vi "Vision_Left_MANUAL_RUN_R0.vi"() -> ()   [LabVIEW 2015]
uses:
  <vilib>/vision/Pattern Matching.llb/IMAQ Curve Parameters.ctl
  <vilib>/vision/Pattern Matching.llb/IMAQ Match Range Setting.ctl
  <vilib>/userdefined/High Color/IMAQdx.ctl
  <vilib>/vision/driver/NI_Vision_Acquisition_Software.lvlib
  <vilib>/vision/NI_Vision_Development_Module.lvlib
panel:
  in  "Range 0 Default\nSetting Values":T1={"Min Scale"=25.0, "Max Scale"=250.0, "Min Score"=850.0, "Lower Transition Scale"=1.0, "Upper Transition Scale"=200.0, "ROI Vertical"=2.0, "ROI Horizontal"=1.0, "Scale Cushion"=15.0, "Curve Parameters"={"Min Length"=15, "Row Search Step"=10, "Col Search Step"=10}, "Beacon Cushion (px)"=3.0, "Max Scale Diff\nfrom Main"=50.0}
  in  "Range 0 Templates":T2={"Sub - 2 File Path"=path "/home/lvuser/Beacon_Templates/Range_0/Range 0.png", "Sub Beacon Template File Path - ARRAY"=[path "/home/lvuser/Beacon_Templates/Range_1/Sub 0 - Range 1.png", path "/home/lvuser/Beacon_Templates/Range_1/Sub 1 - Range 1.png", path "/home/lvuser/Beacon_Templates/Range_1/Sub 2 - Range 1.png", path "/home/lvuser/Beacon_Templates/Range_1/Sub 3 - Range 1.png", path "/home/lvuser/Beacon_Templates/Range_1/Sub 4 - Range 1.png"]}
  in  "Correlation Score Threhsold (Range 0)":sgl=800.0
  in  "stop":bool
  in  "select (true= use advanced features\nfase= dont use)":bool
  in  "Range 3 Default\nSetting Values":T1={"Min Scale"=50.0, "Max Scale"=150.0, "Min Score"=800.0, "Lower Transition Scale"=1.0, "Upper Transition Scale"=120.0, "ROI Vertical"=3.5, "ROI Horizontal"=4.0, "Scale Cushion"=15.0, "Curve Parameters"={"Min Length"=3, "Row Search Step"=5, "Col Search Step"=5}, "Beacon Cushion (px)"=5.0, "Max Scale Diff\nfrom Main"=10.0}
  in  "Range 2 Default\nSetting Values":T1={"Min Scale"=65.0, "Max Scale"=130.0, "Min Score"=800.0, "Lower Transition Scale"=70.0, "Upper Transition Scale"=115.0, "ROI Vertical"=2.8, "ROI Horizontal"=4.0, "Scale Cushion"=2.0, "Curve Parameters"={"Min Length"=10, "Row Search Step"=10, "Col Search Step"=10}, "Beacon Cushion (px)"=15.0, "Max Scale Diff\nfrom Main"=20.0}
  in  "ROI Decay Factor (px)":dbl=50.0
  in  "ROBOT STATE\n(fwd, bwd, neither) 2":i32
  in  "Score Decay \nFactor 2":dbl=50.0
  in  "Range 1 Default\nSetting Values":T1={"Min Scale"=25.0, "Max Scale"=100.0, "Min Score"=800.0, "Lower Transition Scale"=35.0, "Upper Transition Scale"=67.0, "ROI Vertical"=0.75, "ROI Horizontal"=5.0, "Scale Cushion"=23.0, "Curve Parameters"={"Min Length"=15, "Row Search Step"=15, "Col Search Step"=15}, "Beacon Cushion (px)"=25.0, "Max Scale Diff\nfrom Main"=25.0}
  out "Next Template":T3(ring)=enum."Range 0"
  out "Current Template":T3(ring)=enum."Range 0"
  in  "Initial Template":T3(ring)=enum."Range 0"
  in  "Range 3 Templates":T2={"Sub - 2 File Path"=path "/home/lvuser/Beacon_Templates/Range_3/5 Beacons - Range 3.png", "Sub Beacon Template File Path - ARRAY"=[path "/home/lvuser/Beacon_Templates/Range_3/Sub 0 - Range 3.png", path "/home/lvuser/Beacon_Templates/Range_3/Sub 1 - Range 3.png", path "/home/lvuser/Beacon_Templates/Range_3/Sub 2 - Range 3.png", path "/home/lvuser/Beacon_Templates/Range_3/Sub 3 - Range 3.png", path "/home/lvuser/Beacon_Templates/Range_3/Sub 4 - Range 3.png"]}
  in  "Range 2 Templates":T2={"Sub - 2 File Path"=path "/home/lvuser/Beacon_Templates/Range_2/5 Beacons - Range 2.png", "Sub Beacon Template File Path - ARRAY"=[path "/home/lvuser/Beacon_Templates/Range_2/Sub 0 - Range 2.png", path "/home/lvuser/Beacon_Templates/Range_2/Sub 1 - Range 2.png", path "/home/lvuser/Beacon_Templates/Range_2/Sub 2 - Range 2.png", path "/home/lvuser/Beacon_Templates/Range_2/Sub 3 - Range 2.png", path "/home/lvuser/Beacon_Templates/Range_2/Sub 4 - Range 2.png"]}
  in  "Range 1 Templates - LEFT":T2={"Sub - 2 File Path"=path "/home/lvuser/Beacon_Templates/Range_1/2_Beacons_Left - Range 1.png", "Sub Beacon Template File Path - ARRAY"=[path "/home/lvuser/Beacon_Templates/Range_1/Sub 0 - Range 1.png", path "/home/lvuser/Beacon_Templates/Range_1/Sub 1 - Range 1.png", path "/home/lvuser/Beacon_Templates/Range_1/Sub 2 - Range 1.png", path "/home/lvuser/Beacon_Templates/Range_1/Sub 3 - Range 1.png", path "/home/lvuser/Beacon_Templates/Range_1/Sub 4 - Range 1.png"]}
  out "Current Correlation Score":sgl
  in  "Correlation Score Threhsold":sgl=300.0
  out "New Min Score":dbl=850.0
  out "New Low Scale":dbl=50.0
  out "New high Scale":dbl=250.0
  in  "Absolute\nMinimum Score":dbl=750.0
  in  "Absolute\nMaximum Scale":dbl=250.0
  in  "Absolute\nMinimum Scale":dbl=25.0
  in  "Score\nCushion":dbl=192.0
  in  "Avg Scale - Last":dbl=25.73214817047119
  in  "Avg Score - Last":dbl=994.8521728515625
  in  "Max Window\n for Avg":u8=3
  in  "Valid Treshold\nfor Lock":i16=3
  out "Current  Score":sgl
  out "Current  Scale":sgl
  out "Current Valid?":bool
  out "Beacon - Scales":sgl[](array[numeric])
  out "beacon - Scores":sgl[](array[numeric])
  out "Beacons Found":bool[](array[boolean])
  out "Horiztonall Beacon \nCushion (pixels)":sgl=15.0
  out "Tracking Info":T4={"Lock"=FALSE, "Current Valid"=FALSE, "Current Template"=enum."Range 0", "Tracking Coordinates"={"X"=159.0, "Y"=119.0}, "Setting Values"={"Min Score"=850.0, "Min Scale"=50.0, "Max Scale"=250.0, "Curve Parameters"={"Min Length"=15, "Row Search Step"=10, "Col Search Step"=10}}}
  out "dT":u32=467
  out "Avg Scale":dbl=25.73214817047119
  out "Avg Score":dbl=994.8521728515625
  out "Current Search Settings":T7={"Curve Parameters"={"Extraction Mode"=1, "Edge Threshold"=200, "Edge Filter Size"=0, "Min Length"=15, "Row Search Step Size"=10, "Col Search Step Size"=10, "Max Endpoint Gap"=4, "Closed"=TRUE, "Subpixel"=TRUE}, "Match Mode"={"Rotation"=FALSE, "Scale"=TRUE, "Occlusion"=TRUE, "Reserved"=FALSE, "Reserved"=FALSE, "Reserved"=FALSE}, "Range Settings"=[{"Match Constraints"=0, "Min"=-2.0, "Max"=2.0}, {"Match Constraints"=1, "Min"=50.0, "Max"=250.0}, {"Match Constraints"=2, "Min"=0.0, "Max"=20.0}], "Number of Matches"=1, "Minimum Match Score"=850.0, "SubPixel Accuracy"=TRUE, "Adv. Geometric Match Options 2"=[{"Setup Data Item"=20, "Item Value"=0.0}, {"Setup Data Item"=22, "Item Value"=1.0}]} {"Curve Parameters"."Extraction Mode" items=["Normal", "Uniform Regions"]; "Curve Parameters"."Edge Filter Size" items=["Fine", "Normal", "Contour Tracing"]; "Curve Parameters"."Max Endpoint Gap" min=0; "Curve Parameters"."Col Search Step Size" min=1 max=255 step=1; "Curve Parameters"."Row Search Step Size" min=1 max=255 step=1; "Curve Parameters"."Min Length" min=0; "Curve Parameters"."Edge Threshold" min=1 max=350 step=1; "Range Settings"."Max" format="%.2f"; "Range Settings"."Min" format="%.2f"; "Range Settings"."Match Constraints" items=["Rotation Angle (degrees)", "Scale Factor (%)", "Occlusion (%)"]}
  out "Valid Scale History":dbl[](array[numeric]) format="%#_13g"
  out "Valid Score History":dbl[](array[numeric]) format="%#_13g"
  out "Valid Beacon History - in":bool[](array[boolean])
  out "Startup Flag":bool
  out "Lock Status":bool
  out "Y Coordinates":sgl[](array[numeric])
  out "X Coordinates":sgl[](array[numeric])
  out "Right Image out":T8(plugin-control)
  in  "History Size":i32=20
  in  "INITIAL Search Settings":T7={"Curve Parameters"={"Extraction Mode"=1, "Edge Threshold"=200, "Edge Filter Size"=0, "Min Length"=15, "Row Search Step Size"=10, "Col Search Step Size"=10, "Max Endpoint Gap"=4, "Closed"=TRUE, "Subpixel"=TRUE}, "Match Mode"={"Rotation"=FALSE, "Scale"=TRUE, "Occlusion"=TRUE, "Reserved"=FALSE, "Reserved"=FALSE, "Reserved"=FALSE}, "Range Settings"=[{"Match Constraints"=0, "Min"=-2.0, "Max"=2.0}, {"Match Constraints"=1, "Min"=25.0, "Max"=250.0}, {"Match Constraints"=2, "Min"=0.0, "Max"=20.0}], "Number of Matches"=1, "Minimum Match Score"=800.0, "SubPixel Accuracy"=TRUE, "Adv. Geometric Match Options 2"=[{"Setup Data Item"=20, "Item Value"=0.0}, {"Setup Data Item"=22, "Item Value"=1.0}]} {"Curve Parameters"."Extraction Mode" items=["Normal", "Uniform Regions"]; "Curve Parameters"."Edge Filter Size" items=["Fine", "Normal", "Contour Tracing"]; "Curve Parameters"."Max Endpoint Gap" min=0; "Curve Parameters"."Col Search Step Size" min=1 max=255 step=1; "Curve Parameters"."Row Search Step Size" min=1 max=255 step=1; "Curve Parameters"."Min Length" min=0; "Curve Parameters"."Edge Threshold" min=1 max=350 step=1; "Range Settings"."Max" format="%.2f"; "Range Settings"."Min" format="%.2f"; "Range Settings"."Match Constraints" items=["Rotation Angle (degrees)", "Scale Factor (%)", "Occlusion (%)"]; "Adv. Geometric Match Options 2"."Setup Data Item" items=["Curve Extraction Mode", "Curve Edge Threshold", "Curve Edge Filter Size", "Min Curve Length", "Curve Row Search Step Size", "Curve Col Search Step Size", "Curve Max Endpoint Gap", "Extract Closed Curves", "Enable Subpixel Curve Extraction", "Enable Correlation Score", "Enable Subpixel Accuracy", "Subpixel Iterations", "Subpixel Tolerance", "Initial Match List Length", "Enable Target Template Curve Score", "Min Match Separation Distance", "Min Match Separation Angle", "Min Match Separation Scale", "Max Match Overlap", "Enable Coarse Result", "Enable Calibration Support", "Enable Contrast Reversal", "Search Strategy", "Refinement Match Factor", "Subpixel Match Factor"]}
  # "ROI Factore (per Template)"
  # "Template Transition Scales"
  # "Search Parameter Limits"
  # "TEMPLATE FILE PATHS"
  # "Config"
  # "Initial Settings"
  # "test"
  # "Range"
  # "Range"
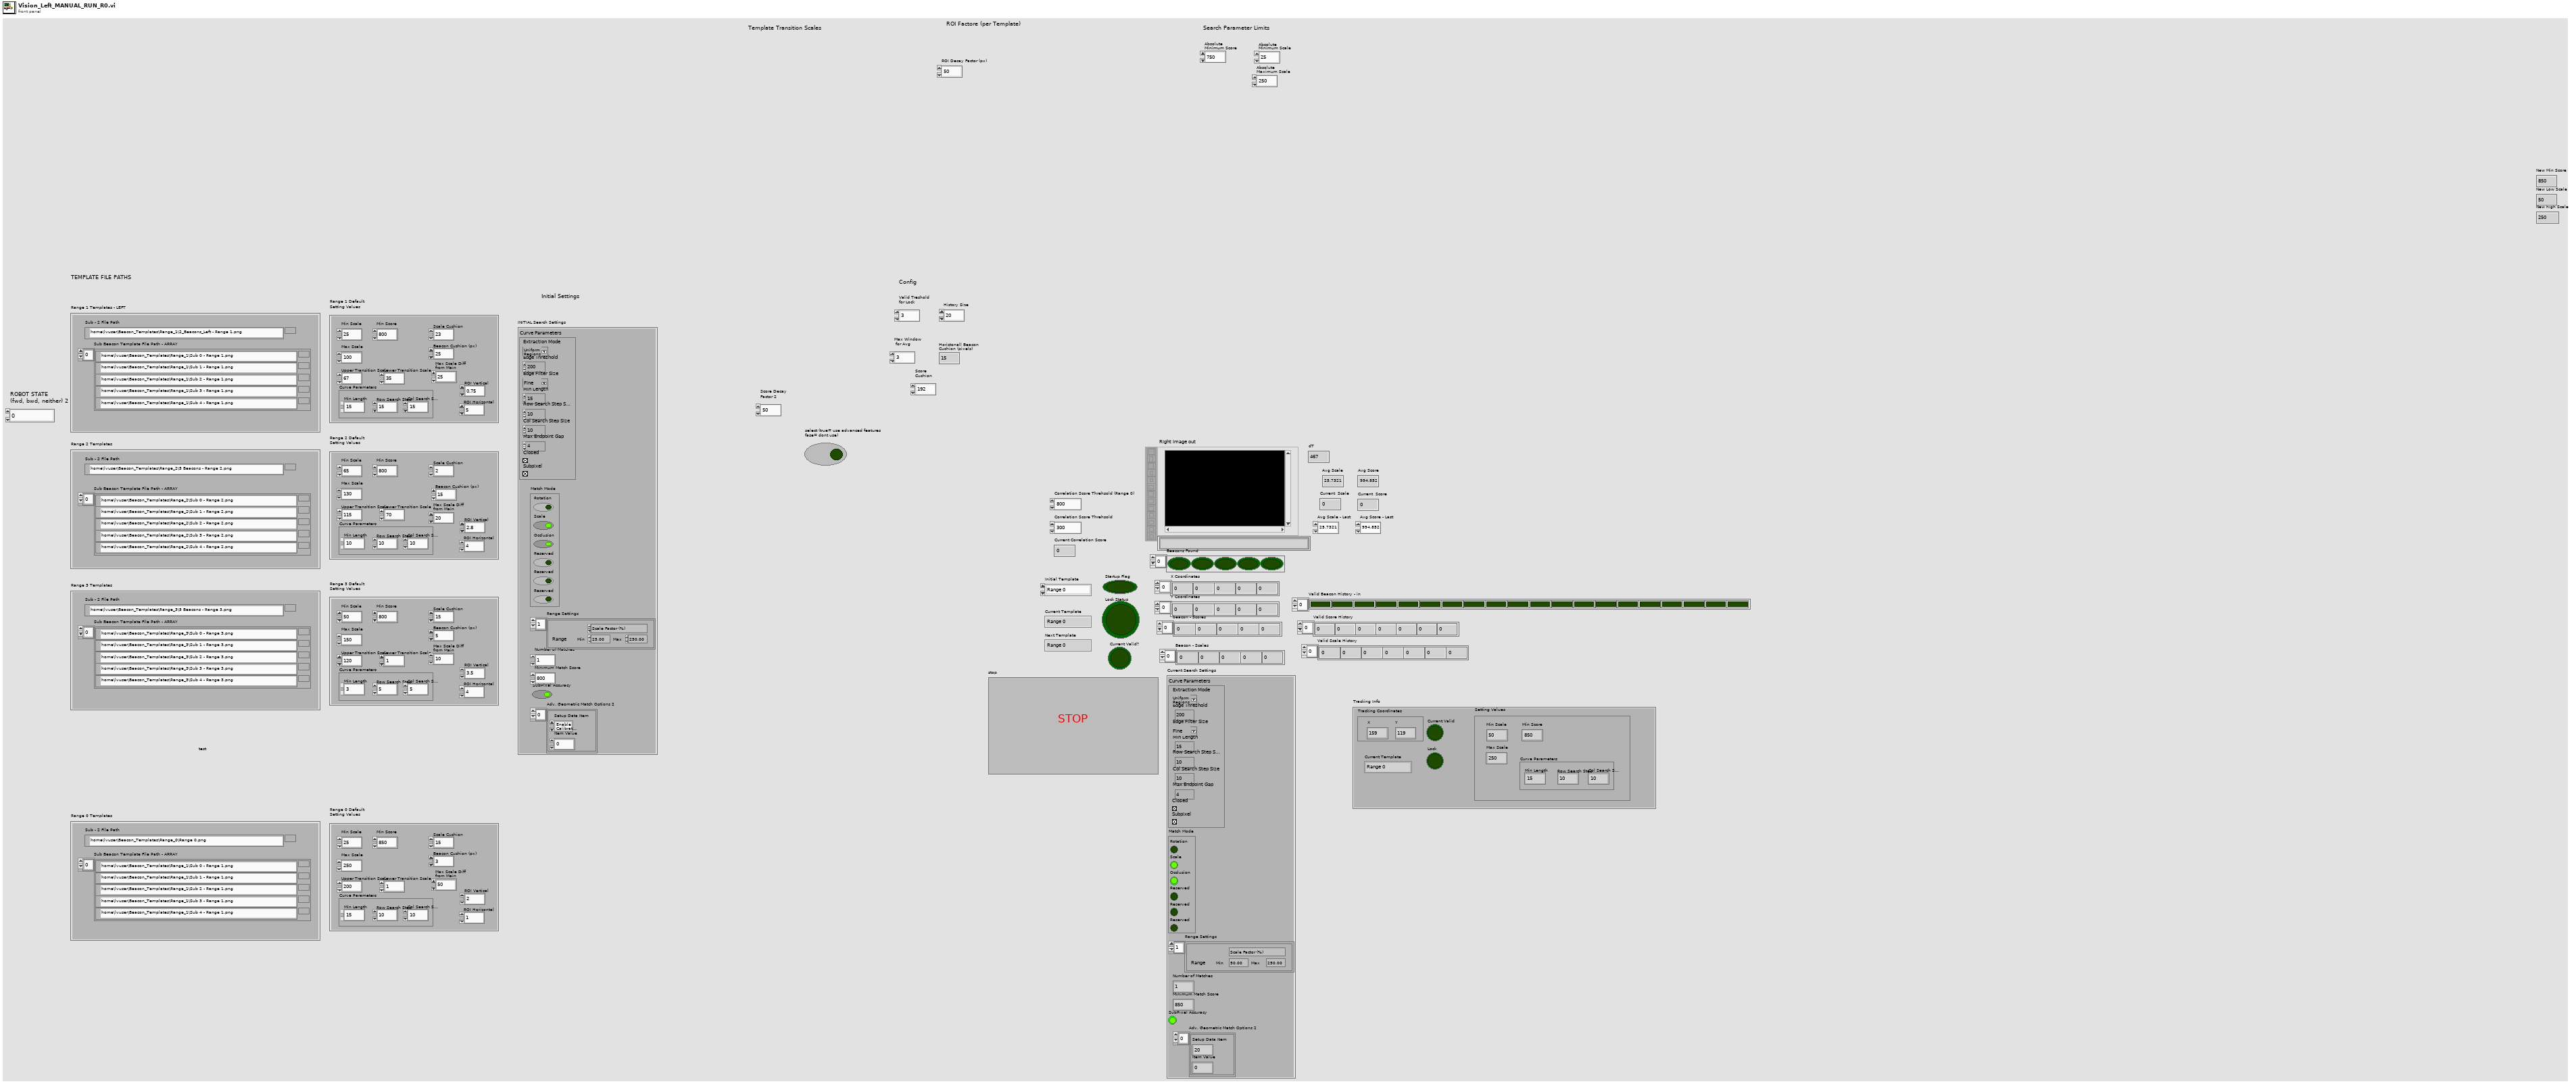
[diagram p1: front panel]
types:
  T1 = cluster{"Min Scale":dbl, "Max Scale":dbl, "Min Score":dbl, "Lower Transition Scale":sgl, "Upper Transition Scale":sgl, "ROI Vertical":dbl, "ROI Horizontal":dbl, "Scale Cushion":dbl, "Curve Parameters":cluster{"Min Length":i32, "Row Search Step":i32, "Col Search Step":i32}, "Beacon Cushion (px)":dbl, "Max Scale Diff\nfrom Main":dbl}
  T2 = cluster{"Sub - 2 File Path":path, "Sub Beacon Template File Path - ARRAY":path[]}
  T3 = enum16{"Range 1", "Range 2", "Range 3", "Range 0"}
  T4 = cluster{"Lock":bool, "Current Valid":bool, "Current Template":enum16{"Range 1", "Range 2", "Range 3", "Range 0"}, "Tracking Coordinates":cluster{"X":dbl, "Y":dbl}, "Setting Values":cluster{"Min Score":dbl, "Min Scale":dbl, "Max Scale":dbl, "Curve Parameters":cluster{"Min Length":i32, "Row Search Step":i32, "Col Search Step":i32}}}
  T5 = typedef "IMAQ Curve Parameters.ctl" = cluster{"Extraction Mode":u32, "Edge Threshold":i32, "Edge Filter Size":u32, "Min Length":i32, "Row Search Step Size":i32, "Col Search Step Size":i32, "Max Endpoint Gap":i32, "Closed":bool, "Subpixel":bool}
  T6 = typedef "IMAQ Match Range Setting.ctl" = cluster{"Match Constraints":u32, "Min":dbl, "Max":dbl}
  T7 = cluster{"Curve Parameters":T5, "Match Mode":cluster{"Rotation":bool, "Scale":bool, "Occlusion":bool, "Reserved":bool, "Reserved":bool, "Reserved":bool}, "Range Settings":T6[], "Number of Matches":i32, "Minimum Match Score":sgl, "SubPixel Accuracy":bool, "Adv. Geometric Match Options 2":cluster{"Setup Data Item":u16, "Item Value":dbl}[]}
  T8 = typedef "IMAQ Image.ctl" = refnum<image>
  T9 = typedef "IMAQdx.ctl" = refnum<k21>
  T10 = typedef "Image Type" = u32
  T11 = typedef "ROI Descriptor" = cluster{"Global Rectangle":i32[], "Contours":cluster{"ID":enum32{"External", "Internal"}, "Type":u32, "Coordinates":i32[]}[]}
  T12 = typedef "IMAQ GM Match Report.ctl" = cluster{"Position":cluster{"x":sgl, "y":sgl}, "Angle":sgl, "Scale":sgl, "Score":sgl, "Bounding Box":cluster{"x":sgl, "y":sgl}[], "Contrast Reversed":bool, "Occlusion %":sgl, "Template Target Curve Score":sgl, "Target Template Curve Score":sgl, "Correlation Score":sgl}
  T13 = cluster{"Matches[0]":T12, "Matches[1]":T12, "Matches[2]":T12, "Matches[3]":T12, "Matches[4]":T12, "Matches[5]":T12, "Matches[6]":T12, "Matches[7]":T12, "Matches[8]":T12}
  T14 = cluster{"Bounding Box[0]":cluster{"x":sgl, "y":sgl}, "Bounding Box[1]":cluster{"x":sgl, "y":sgl}, "Bounding Box[2]":cluster{"x":sgl, "y":sgl}, "Bounding Box[3]":cluster{"x":sgl, "y":sgl}, "Bounding Box[4]":cluster{"x":sgl, "y":sgl}, "Bounding Box[5]":cluster{"x":sgl, "y":sgl}, "Bounding Box[6]":cluster{"x":sgl, "y":sgl}, "Bounding Box[7]":cluster{"x":sgl, "y":sgl}, "Bounding Box[8]":cluster{"x":sgl, "y":sgl}}
  T15 = cluster{"Matches (Geometric Matching 1)[0]":T12, "Matches (Geometric Matching 1)[1]":T12, "Matches (Geometric Matching 1)[2]":T12, "Matches (Geometric Matching 1)[3]":T12, "Matches (Geometric Matching 1)[4]":T12, "Matches (Geometric Matching 1)[5]":T12, "Matches (Geometric Matching 1)[6]":T12, "Matches (Geometric Matching 1)[7]":T12, "Matches (Geometric Matching 1)[8]":T12}
  T16 = cluster{"Min Length":i32, "Row Search Step":i32, "Col Search Step":i32}
  T17 = cluster{"Extraction Mode":u32, "Edge Threshold":i32, "Edge Filter Size":u32, "Min Length":i32, "Row Search Step":i32, "Col Search Step":i32, "Max Endpoint Gap":i32, "Closed":bool, "Subpixel":bool}
  T18 = typedef "IMAQ Rectangle" = cluster{"Left":i32, "Top":i32, "Right":i32, "Bottom":i32, "Rotation":dbl}
  T19 = cluster{"Min Length":i32, "Row Search Step Size":i32, "Col Search Step Size":i32}
  T20 = cluster{"Min Score":dbl, "Min":dbl, "Max":dbl, cluster{"Min Length":i32, "Row Search Step Size":i32, "Col Search Step Size":i32}}
  T21 = cluster{bool, bool, "Initial Template":enum16{"Range 1", "Range 2", "Range 3", "Range 0"}, "Position":cluster{"x":dbl, "y":dbl}, cluster{"Min Score":dbl, "Min":dbl, "Max":dbl, cluster{"Min Length":i32, "Row Search Step Size":i32, "Col Search Step Size":i32}}}
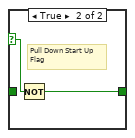
[diagram p2: hidden frame]
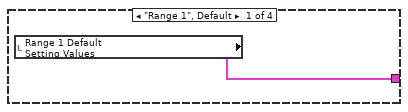
[diagram p3: hidden frame]
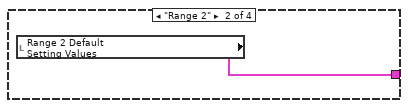
[diagram p4: hidden frame]
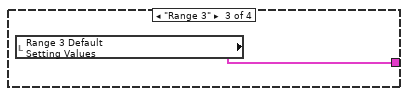
[diagram p5: hidden frame]
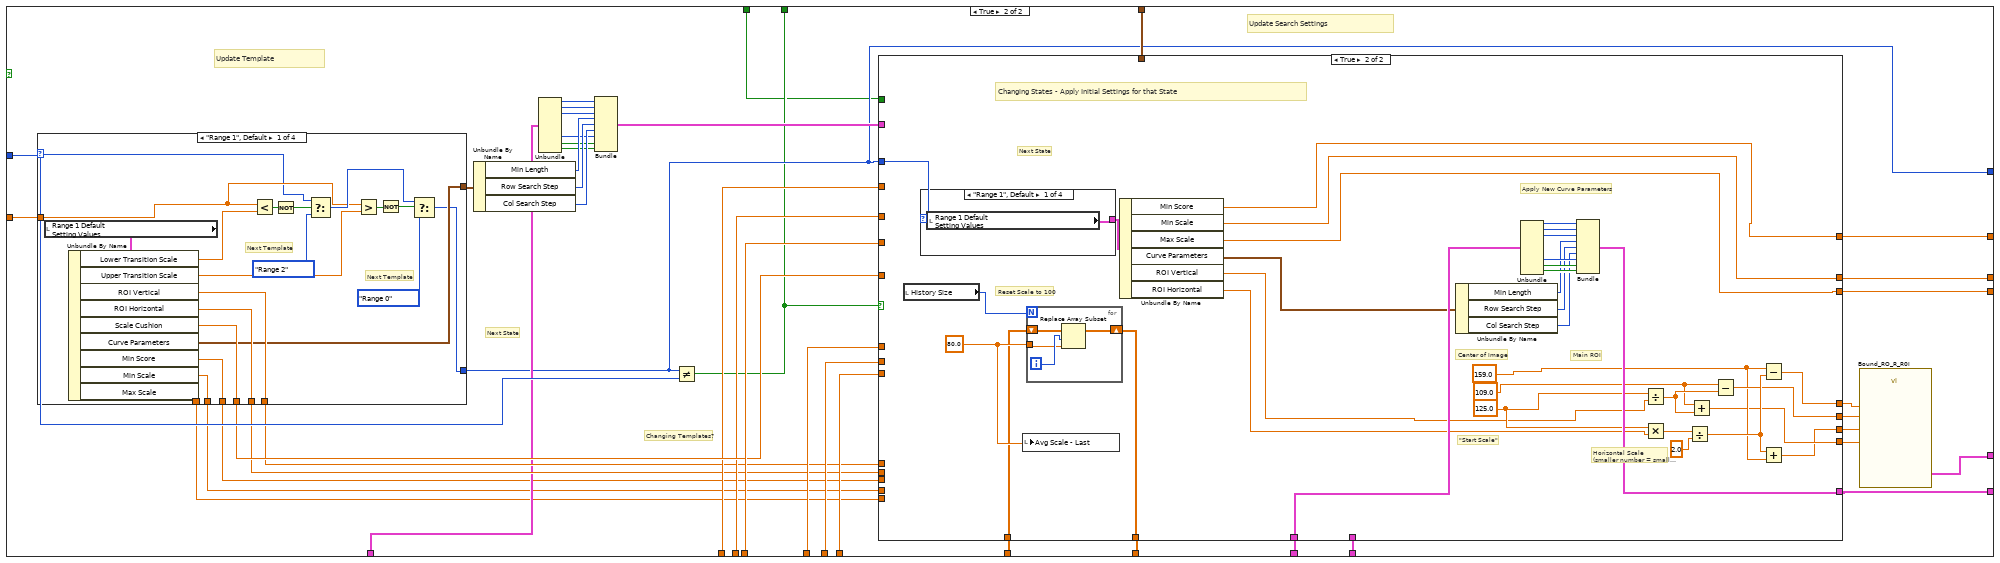
[diagram p6: hidden frame]
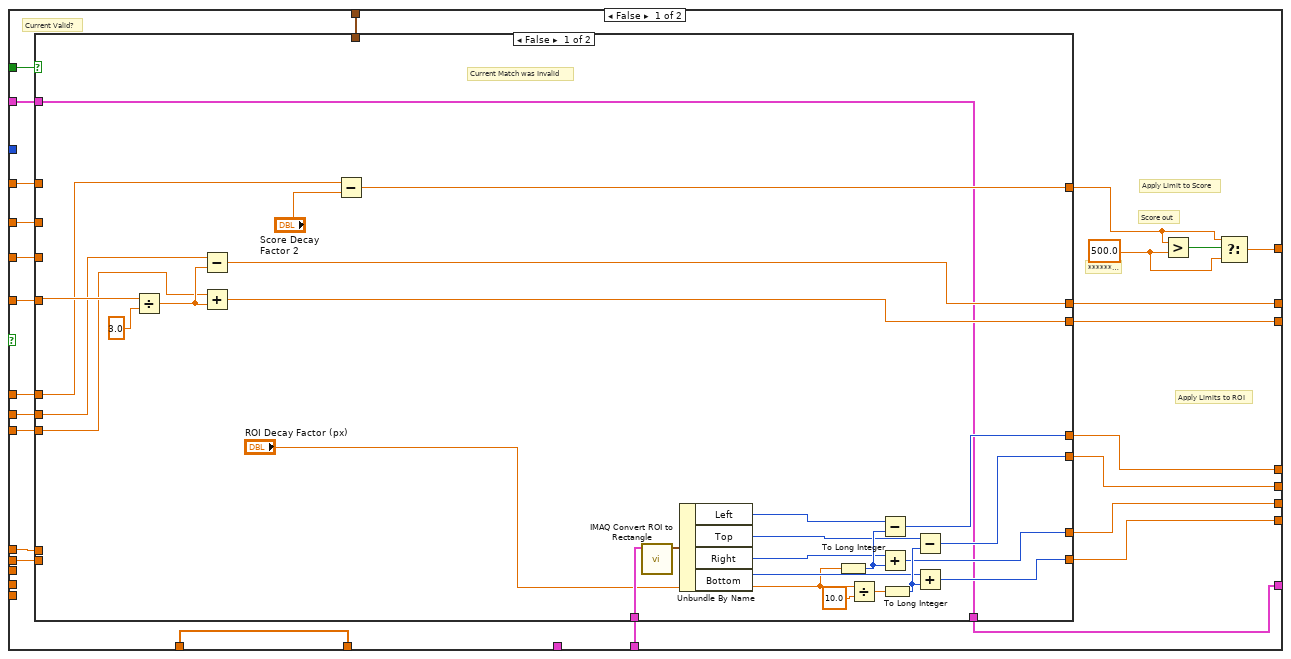
[diagram p7: hidden frame]
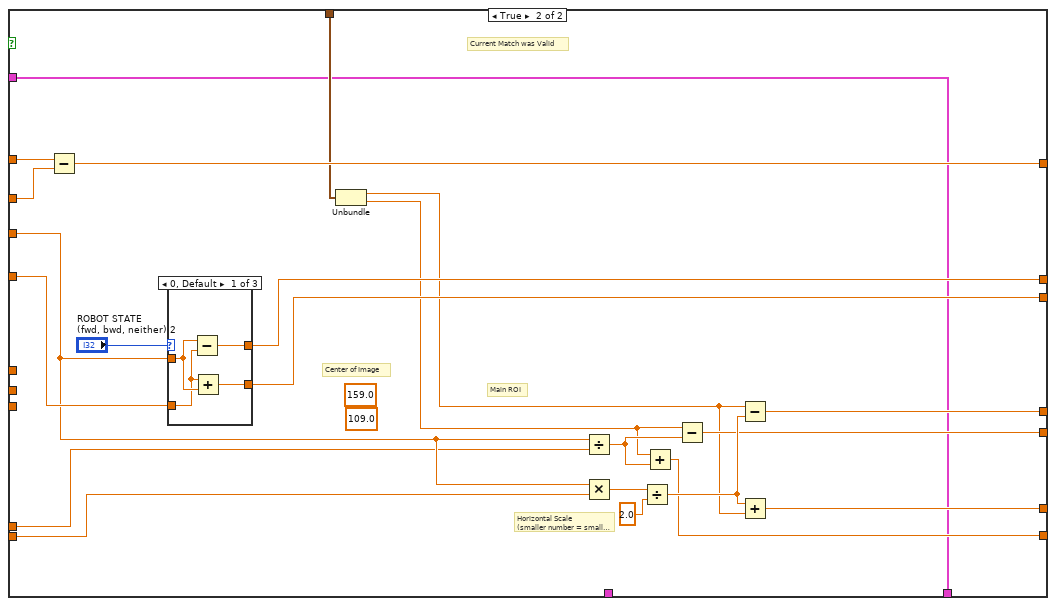
[diagram p8: hidden frame]
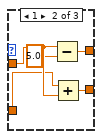
[diagram p9: hidden frame]
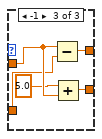
[diagram p10: hidden frame]
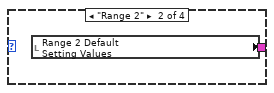
[diagram p11: hidden frame]
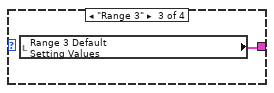
[diagram p12: hidden frame]
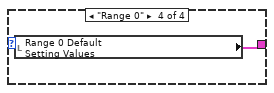
[diagram p13: hidden frame]
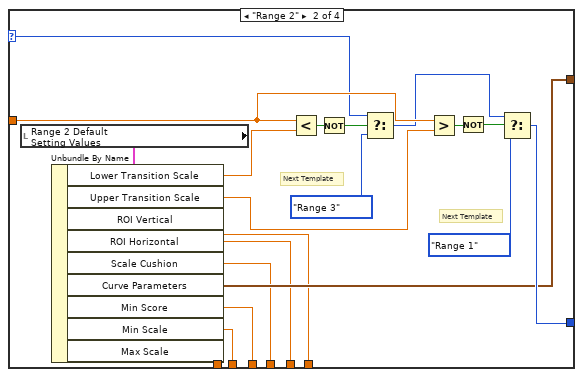
[diagram p14: hidden frame]
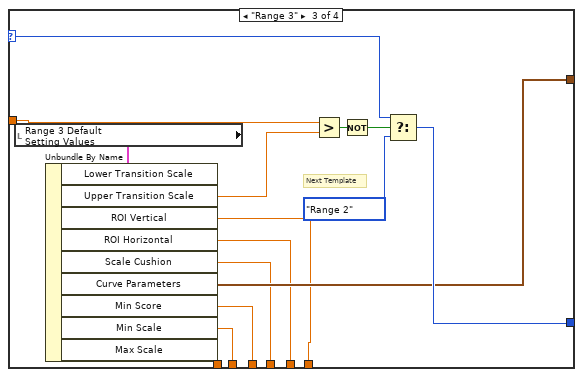
[diagram p15: hidden frame]
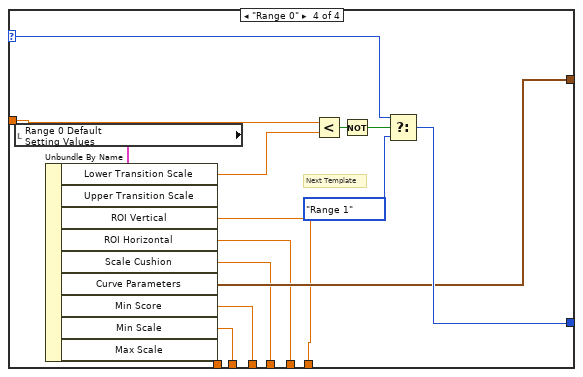
[diagram p16: hidden frame]
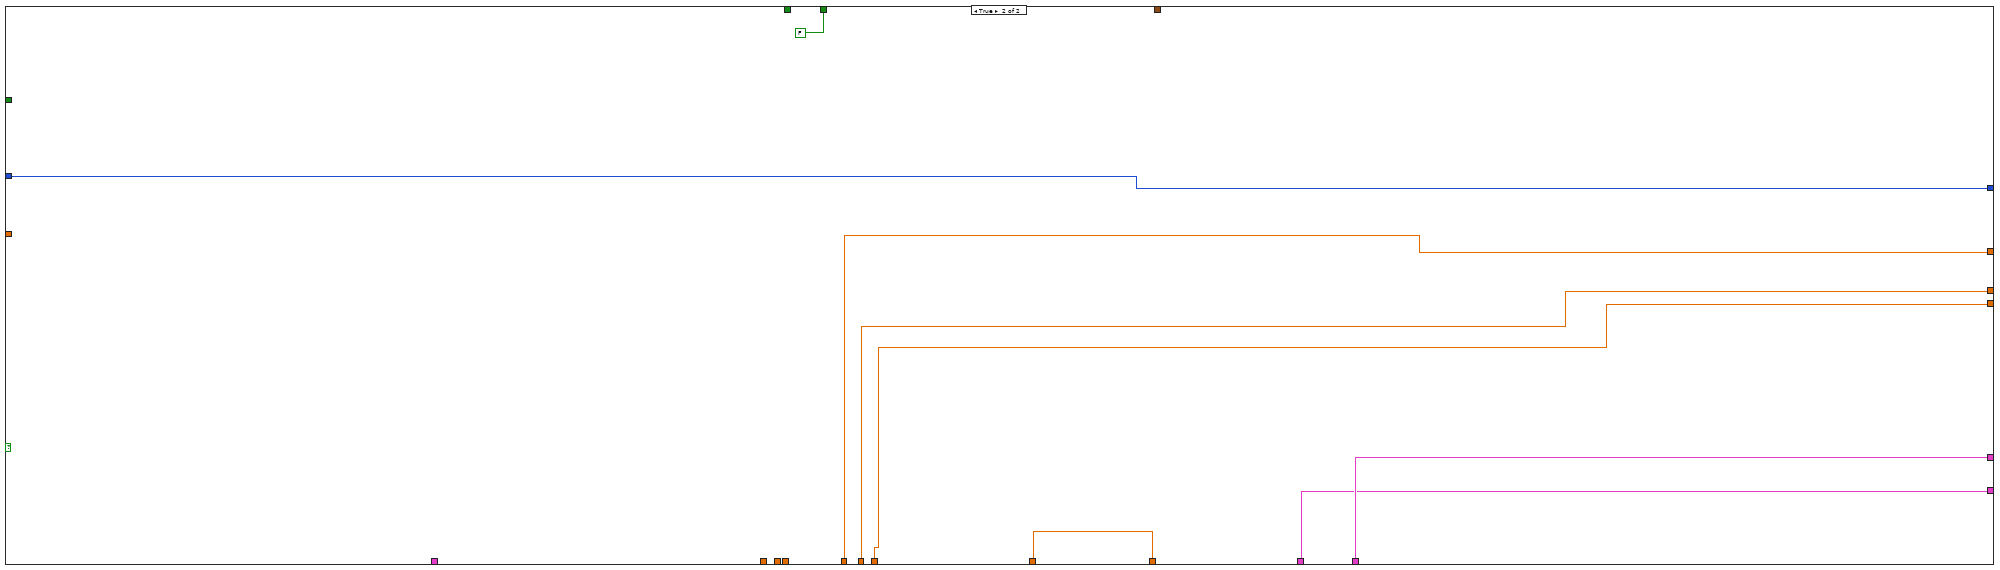
[diagram p17: hidden frame]
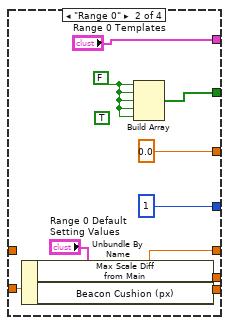
[diagram p18: hidden frame]
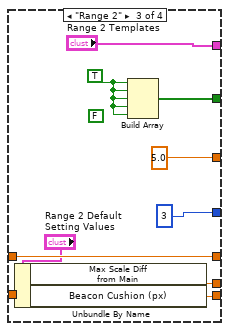
[diagram p19: hidden frame]
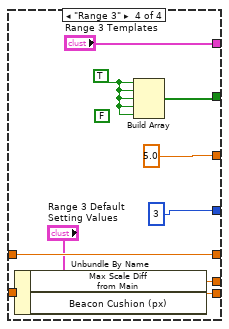
[diagram p20: hidden frame]
diagram:
  n1 = flat-sequence {
    tunnel: [w38] -> w16
    tunnel: ["INITIAL Search Settings"] -> w15
    tunnel: ["Initial Template"] -> w14
    tunnel: [TRUE] -> w13
    tunnel: [w35] -> w12
    tunnel: [w34] -> w11
    tunnel: [w33] -> w10
    tunnel: [w32] -> w9
    tunnel: [w31] -> w8
    tunnel: ["History Size"] -> w7
    tunnel: [750.0] -> w6
    tunnel: [100.0] -> w5
    tunnel: [w19] -> w4
    tunnel: [w18] -> w3
    tunnel: [w17] -> w2
    tunnel: w16 -> [w64]
    tunnel: w15 -> [w63]
    tunnel: w14 -> [w62]
    tunnel: w13 -> [w61]
    tunnel: w12 -> [w57]
    tunnel: w11 -> [w54]
    tunnel: w10 -> [w60]
    tunnel: w9 -> [w59]
    tunnel: w8 -> [w58]
    tunnel: w7 -> [w56]
    tunnel: w6 -> [_]
    tunnel: w5 -> [_]
    tunnel: w4 -> [w53]
    tunnel: w3 -> [w52]
    tunnel: w2 -> [w51]
    tunnel: [w50] -> w1
    tunnel: w1 -> [w819]
    frame #0 {
      w24 = "[NIIMAQ_HEADER]\nType = 2\nVersion = 8\n\n[CAMERA_DATA]\nAcquisitionAttributes::Bayer::Algorithm = \"Bilinear\"\nAcquisitionAttributes::Bayer::GainB = \"1\"\nAcquisitionAttributes::Bayer::GainG = \"1\"\nAcquisitionAttributes::Bayer::GainR = \"1\"\nAcquisitionAttributes::Bayer::Pattern = \"Use hardware value\"\nAcquisitionAttributes::BitsPerPixel = \"Use hardware value\"\nAcquisitionAttributes::IgnoreFirstFrame = \"false\"\nAcquisitionAttributes::ImageDecoderCopyMode = \"Auto\"\nAcquisitionAttributes::OutputImageType = \"Auto\"\nAcquisitionAttributes::OverwriteMode = \"Get Newest\"\nAcquisitionAttributes::PixelSignedness = \"Use hardware value\"\nAcquisitionAttributes::ReceiveTimestampMode = \"None\"\nAcquisitionAttributes::ShiftPixelBits = \"false\"\nAcquisitionAttributes::SwapPixelBytes = \"false\"\nAcquisitionAttributes::Timeout = \"5000\"\nAcquisitionAttributes::VerticalMirror = \"false\"\nAcquisitionAttributes::VideoMode = \"320x240 YUY2 30.00fps\"\nCameraAttributes::BacklightCompensation::Mode = \"Manual\"\nCameraAttributes::BacklightCompensation::Value = \"false\"\nCameraAttributes::Brightness::Mode = \"UnknownEnumValue\"\nCameraAttributes::Brightness::Value = \"133\"\nCameraAttributes::Contrast::Mode = \"Manual\"\nCameraAttributes::Contrast::Value = \"0\"\nCameraAttributes::Exposure::Mode = \"Auto\"\nCameraAttributes::Focus::Mode = \"Auto\"\nCameraAttributes::Pan::Mode = \"Manual\"\nCameraAttributes::Pan::Value = \"0\"\nCameraAttributes::Saturation::Mode = \"Manual\"\nCameraAttributes::Saturation::Value = \"103\"\nCameraAttributes::Sharpness::Mode = \"Manual\"\nCameraAttributes::Sharpness::Value = \"25\"\nCameraAttributes::Tilt::Mode = \"Manual\"\nCameraAttributes::Tilt::Value = \"0\"\nCameraAttributes::WhiteBalance::Mode = \"Auto\"\nCameraAttributes::Zoom::Mode = \"Manual\"\nCameraAttributes::Zoom::Value = \"0\"\n"  # Attributes
      w45 = T10 0 items=["Grayscale (U8)", "Grayscale (I16)", "Grayscale (SGL)", "Complex (CSG)", "RGB (U32)", "HSL (U32)", "RGB (U64)", "Grayscale (U16)"] ("Image Type")
      # "avg start scale"
      # "Score History"
      # "Scale History"
      # "Valid Match History\n(main beacon)"
      # "Template State"
      # "Search Parameters"
      # "StartUp = True"
      # "Initial ROI Descriptor"
      # "INITIALIZE"
      n2 = call <vilib>:"IMAQdx Open Camera.vi"("Session In"=T9 "cam0") -> ("error out"=w22:errorcluster, "Session Out"=w23:T9)  [unwired: 2 in, 7 out]
      n3 = call <vilib>:"IMAQdx Read Attributes From String.vi"("error in"=w22, "Attributes String In"=w24, "Session In"=w23) -> ("error out"=w21:errorcluster, "Session Out"=w20:T9)  [unwired: 7 out]
      n4 = Bundle(0, 0, 640, 480, 0) -> (w44:cluster{i32, i32, i32, i32, i32})  [unwired: 1 in]
      n5 = call "IMAQ Convert Rectangle to ROI"("Rectangle"=w44) -> ("ROI Descriptor"=w38:T11)  [unwired: 8 in, 1 out]
      n6 = call "IMAQ Create"("Image Name"="Left_Image", "Image Type"=w45) -> ("New Image"=w35:T8, "error out"=w34:errorcluster)  [unwired: 3 in]
      n7 = Initialize Array(FALSE, "History Size") -> (w33:bool[])
      n8 = Initialize Array(0.0, "History Size") -> (w31:dbl[])
      n9 = Initialize Array(0.0, "History Size") -> (w32:dbl[])
      n10 = call <vilib>:"IMAQdx Configure Grab.vi"("error in"=w21, "Session In"=w20) -> ("error out"=w17:errorcluster, "Session Out"=w19:T9)  [unwired: 8 in]
      n11 = call "IMAQ Create"("Image Name"="Original") -> ("New Image"=w18:T8)  [unwired: 4 in, 1 out]
    }
    frame #1 {
      # "Avg Scale"
      # "Avg Score"
      # "Score History"
      # "Scale History"
      # "Valid Match History\n(main beacon)"
      # "Sub Beacon Search Array"
      # "StartUp = True"
      # "Template State"
      # "Search Parameters"
      # "ROI"
      n12 = call "Tick Count"() -> ("Tick Count(mSec)"=w55:u32)
      n13 = while {
        shift-right: [w77] -> _
        shift-left: w64 -> [w91]
        shift-right: [w87] -> _
        shift-left: w63 -> [w92]
        shift-right: [w76] -> _
        shift-left: w62 -> [w79]
        shift-right: [w74] -> _
        shift-left: w61 -> [w75]
        shift-right: [w83] -> _
        shift-left: w60 -> [w84]
        shift-right: [w73] -> _
        shift-left: w59 -> [w82]
        shift-right: [w80] -> _
        shift-left: w58 -> [w81]
        shift-right: [w86] -> _
        shift-left: w57 -> [w93]
        tunnel: w56 -> [w98]
        shift-right: [w96] -> _
        shift-left: w55 -> [w97]
        tunnel: w54 -> [w85]
        tunnel: w53 -> [w72]
        tunnel: w52 -> [w71]
        tunnel: w51 -> [w70]
        tunnel: [w67] -> w50
        stop <- "stop" stop-if-true
        n14 = call "Tick Count2"() -> ("Tick Count(mSec)"=w96:u32)
        n15 = Subtract(x=w96, y=w97) -> (x-y=→"dT":u32)
        n16 = flat-sequence {
          tunnel: [w106] -> w89
          tunnel: [w105] -> w94
          tunnel: w93 -> [w105]
          tunnel: [w105] -> w86
          tunnel: w85 -> [_]
          tunnel: w72 -> [w104]
          tunnel: w71 -> [w103]
          tunnel: w70 -> [w102]
          tunnel: [w101] -> w69
          tunnel: [w100] -> w68
          tunnel: [w99] -> w66
          tunnel: w79 -> [w111]
          tunnel: w84 -> [w223]
          tunnel: w82 -> [w222]
          tunnel: w81 -> [w221]
          tunnel: w98 -> [_]
          tunnel: w94 -> [w122]
          tunnel: w92 -> [w123]
          tunnel: w91 -> [w125]
          tunnel: [w190] -> w90
          tunnel: w89 -> [w179]
          tunnel: [w179] -> w88
          tunnel: [w178] -> w83
          tunnel: [w147] -> _
          tunnel: [w177] -> w80
          tunnel: w75 -> [w144]
          tunnel: [w107] -> w78
          tunnel: [w149] -> w77
          tunnel: [w107] -> w76
          tunnel: [w143] -> w74
          tunnel: [w148] -> w73
          tunnel: w69 -> [w117]
          tunnel: w68 -> [w116]
          tunnel: [w115] -> w67
          tunnel: w66 -> [w115]
          tunnel: w90 -> [w816]
          tunnel: w88 -> [w817]
          tunnel: [w816] -> w87
          tunnel: [w815] -> _
          tunnel: w78 -> [w815]
          frame #0 {
            # "Aquire Image"
            n17 = shared-variable "RT myRIO Target - Overlord\\Localization_Variables_r0.lvlib\\Left Servo Angle_Current"() -> (w106:dbl)  [unwired: 1 in, 1 out]
            n18 = call <vilib>:"IMAQdx Grab2.vi"("error in"=w102, "Image In"=w103, "Session In"=w104) -> ("error out"=w100:errorcluster, "Image Out"=w101:T8, "Session Out"=w99:T9)  [unwired: 5 in, 1 out]
          }
          frame #1 {
            w107 = T3."Range 0" ("Initial Template")
            (unwired) T3."Range 1" ("Initial Template 2")
            w135 = 6 items=["Red", "Green", "Blue", "Hue", "Saturation", "Luminance", "Value", "Intensity"] ("Color Plane")
            w193 = u32 1 ("index")
            # "Tracking Position"
            # "ROI center"
            # "Add mode when CLose to look for all individual beacons with full ROI"
            # "Service Start Up Flag"
            # "Change States?"
            # "Next Template"
            # "Max Scale"
            # "Min Scale"
            # "Min Score"
            # "Curve p"
            # "ROI"
            # "Current Scale Range"
            # "Current Min Score"
            # "Avg Score"
            # "Avg Scale"
            # "Startup?"
            # "********** Look into False case **********"
            # "SUm # of Sub-Beacons Found, Check if Enoough\nto be considered Valid"
            # "Update Tracking Coordinates"
            # "Next Settings"
            # "Current Settings"
            # "Current Min\n& Max Scale"
            # "Scale"
            # "Min Score"
            # "Lower Scale"
            # "Upper Scale"
            # "Min Score out"
            # "Score History"
            # "Min Required to use avarage"
            # "Scale History"
            # "History Size"
            # "Calculate Average Score/Scale"
            # "****# of previous in history that must be true\nin order for position to be considered \"locked\""
            # "Scale History"
            # "Score History"
            # "Valid History"
            # "Update History Data"
            # "1 Match FOund?"
            # "# of Sub Beacons"
            # "Sub Beacons to Search For"
            # "# Sub Beacons to Find in\norder to be valid"
            # "Template Filepath & Sub Beacon Array"
            # "Select Current Template Config"
            # "Pattern Match to Current Template"
            # "Apply FIltering"
            n19 = call "IMAQ ImageBorderSize"("Get/Set Status? (Set)"=TRUE, "Image"=w117, "Image border size in"=13 ("Border Size"), "error in (no error)"=w116) -> ("Image Out"=w134:T8, "error out"=w138:errorcluster)  [unwired: 1 out]
            n20 = call "IMAQ ExtractSingleColorPlane"("Color Plane"=w135, "error in (no error)"=w138, "Image Src"=w134) -> ("error out"=w133:errorcluster, "Image Dst Out"=w131:T8)  [unwired: 1 in, 6 out]
            n21 = call "IMAQ Convolute"("Kernel"=sgl[][] [[1.0, 2.0, 1.0], [2.0, 4.0, 2.0], [1.0, 2.0, 1.0]], "Divider (kernel sum)"=sgl 9.0 ("Divider"), "error in (no error)"=w133, "Image Src"=w131) -> ("error out"=w130:errorcluster, "Image Dst Out"=w127:T8)  [unwired: 3 in, 3 out]
            n22 = call "IMAQ Convolute"("Kernel"=sgl[][] [[-1.0, -1.0, -1.0, -1.0, -1.0, -1.0, -1.0, -1.0, -1.0, -1.0, -1.0, -1.0, -1.0, -1.0, -1.0, -1.0, -1.0, -1.0, -1.0, -1.0, -1.0, -1.0, -1.0, -1.0, -1.0, -1.0, -1.0], [-1.0, -1.0, -1.0, -1.0, -1.0, -1.0, -1.0, -1.0, -1.0, -1.0, -1.0, -1.0, -1.0, -1.0, -1.0, -1.0, -1.0, -1.0, -1.0, -1.0, -1.0, -1.0, -1.0, -1.0, -1.0, -1.0, -1.0], [-1.0, -1.0, -1.0, -1.0, -1.0, -1.0, -1.0, -1.0, -1.0, -1.0, -1.0, -1.0, -1.0, -1.0, -1.0, -1.0, -1.0, -1.0, -1.0, -1.0, -1.0, -1.0, -1.0, -1.0, -1.0, -1.0, -1.0], [-1.0, -1.0, -1.0, -1.0, -1.0, -1.0, -1.0, -1.0, -1.0, -1.0, -1.0, -1.0, -1.0, -1.0, -1.0, -1.0, -1.0, -1.0, -1.0, -1.0, -1.0, -1.0, -1.0, -1.0, -1.0, -1.0, -1.0], [-1.0, -1.0, -1.0, -1.0, -1.0, -1.0, -1.0, -1.0, -1.0, -1.0, -1.0, -1.0, -1.0, -1.0, -1.0, -1.0, -1.0, -1.0, -1.0, -1.0, -1.0, -1.0, -1.0, -1.0, -1.0, -1.0, -1.0], [-1.0, -1.0, -1.0, -1.0, -1.0, -1.0, -1.0, -1.0, -1.0, -1.0, -1.0, -1.0, -1.0, -1.0, -1.0, -1.0, -1.0, -1.0, -1.0, -1.0, -1.0, -1.0, -1.0, -1.0, -1.0, -1.0, -1.0], [-1.0, -1.0, -1.0, -1.0, -1.0, -1.0, -1.0, -1.0, -1.0, -1.0, -1.0, -1.0, -1.0, -1.0, -1.0, -1.0, -1.0, -1.0, -1.0, -1.0, -1.0, -1.0, -1.0, -1.0, -1.0, -1.0, -1.0], [-1.0, -1.0, -1.0, -1.0, -1.0, -1.0, -1.0, -1.0, -1.0, -1.0, -1.0, -1.0, -1.0, -1.0, -1.0, -1.0, -1.0, -1.0, -1.0, -1.0, -1.0, -1.0, -1.0, -1.0, -1.0, -1.0, -1.0], [-1.0, -1.0, -1.0, -1.0, -1.0, -1.0, -1.0, -1.0, -1.0, -1.0, -1.0, -1.0, -1.0, -1.0, -1.0, -1.0, -1.0, -1.0, -1.0, -1.0, -1.0, -1.0, -1.0, -1.0, -1.0, -1.0, -1.0], [-1.0, -1.0, -1.0, -1.0, -1.0, -1.0, -1.0, -1.0, -1.0, -1.0, -1.0, -1.0, -1.0, -1.0, -1.0, -1.0, -1.0, -1.0, -1.0, -1.0, -1.0, -1.0, -1.0, -1.0, -1.0, -1.0, -1.0], [-1.0, -1.0, -1.0, -1.0, -1.0, -1.0, -1.0, -1.0, -1.0, -1.0, -1.0, -1.0, -1.0, -1.0, -1.0, -1.0, -1.0, -1.0, -1.0, -1.0, -1.0, -1.0, -1.0, -1.0, -1.0, -1.0, -1.0], [-1.0, -1.0, -1.0, -1.0, -1.0, -1.0, -1.0, -1.0, -1.0, -1.0, -1.0, -1.0, -1.0, -1.0, -1.0, -1.0, -1.0, -1.0, -1.0, -1.0, -1.0, -1.0, -1.0, -1.0, -1.0, -1.0, -1.0], [-1.0, -1.0, -1.0, -1.0, -1.0, -1.0, -1.0, -1.0, -1.0, -1.0, -1.0, -1.0, -1.0, -1.0, -1.0, -1.0, -1.0, -1.0, -1.0, -1.0, -1.0, -1.0, -1.0, -1.0, -1.0, -1.0, -1.0], [-1.0, -1.0, -1.0, -1.0, -1.0, -1.0, -1.0, -1.0, -1.0, -1.0, -1.0, -1.0, -1.0, 728.0, -1.0, -1.0, -1.0, -1.0, -1.0, -1.0, -1.0, -1.0, -1.0, -1.0, -1.0, -1.0, -1.0], [-1.0, -1.0, -1.0, -1.0, -1.0, -1.0, -1.0, -1.0, -1.0, -1.0, -1.0, -1.0, -1.0, -1.0, -1.0, -1.0, -1.0, -1.0, -1.0, -1.0, -1.0, -1.0, -1.0, -1.0, -1.0, -1.0, -1.0], [-1.0, -1.0, -1.0, -1.0, -1.0, -1.0, -1.0, -1.0, -1.0, -1.0, -1.0, -1.0, -1.0, -1.0, -1.0, -1.0, -1.0, -1.0, -1.0, -1.0, -1.0, -1.0, -1.0, -1.0, -1.0, -1.0, -1.0], [-1.0, -1.0, -1.0, -1.0, -1.0, -1.0, -1.0, -1.0, -1.0, -1.0, -1.0, -1.0, -1.0, -1.0, -1.0, -1.0, -1.0, -1.0, -1.0, -1.0, -1.0, -1.0, -1.0, -1.0, -1.0, -1.0, -1.0], [-1.0, -1.0, -1.0, -1.0, -1.0, -1.0, -1.0, -1.0, -1.0, -1.0, -1.0, -1.0, -1.0, -1.0, -1.0, -1.0, -1.0, -1.0, -1.0, -1.0, -1.0, -1.0, -1.0, -1.0, -1.0, -1.0, -1.0], [-1.0, -1.0, -1.0, -1.0, -1.0, -1.0, -1.0, -1.0, -1.0, -1.0, -1.0, -1.0, -1.0, -1.0, -1.0, -1.0, -1.0, -1.0, -1.0, -1.0, -1.0, -1.0, -1.0, -1.0, -1.0, -1.0, -1.0], [-1.0, -1.0, -1.0, -1.0, -1.0, -1.0, -1.0, -1.0, -1.0, -1.0, -1.0, -1.0, -1.0, -1.0, -1.0, -1.0, -1.0, -1.0, -1.0, -1.0, -1.0, -1.0, -1.0, -1.0, -1.0, -1.0, -1.0], [-1.0, -1.0, -1.0, -1.0, -1.0, -1.0, -1.0, -1.0, -1.0, -1.0, -1.0, -1.0, -1.0, -1.0, -1.0, -1.0, -1.0, -1.0, -1.0, -1.0, -1.0, -1.0, -1.0, -1.0, -1.0, -1.0, -1.0], [-1.0, -1.0, -1.0, -1.0, -1.0, -1.0, -1.0, -1.0, -1.0, -1.0, -1.0, -1.0, -1.0, -1.0, -1.0, -1.0, -1.0, -1.0, -1.0, -1.0, -1.0, -1.0, -1.0, -1.0, -1.0, -1.0, -1.0], [-1.0, -1.0, -1.0, -1.0, -1.0, -1.0, -1.0, -1.0, -1.0, -1.0, -1.0, -1.0, -1.0, -1.0, -1.0, -1.0, -1.0, -1.0, -1.0, -1.0, -1.0, -1.0, -1.0, -1.0, -1.0, -1.0, -1.0], [-1.0, -1.0, -1.0, -1.0, -1.0, -1.0, -1.0, -1.0, -1.0, -1.0, -1.0, -1.0, -1.0, -1.0, -1.0, -1.0, -1.0, -1.0, -1.0, -1.0, -1.0, -1.0, -1.0, -1.0, -1.0, -1.0, -1.0], [-1.0, -1.0, -1.0, -1.0, -1.0, -1.0, -1.0, -1.0, -1.0, -1.0, -1.0, -1.0, -1.0, -1.0, -1.0, -1.0, -1.0, -1.0, -1.0, -1.0, -1.0, -1.0, -1.0, -1.0, -1.0, -1.0, -1.0], [-1.0, -1.0, -1.0, -1.0, -1.0, -1.0, -1.0, -1.0, -1.0, -1.0, -1.0, -1.0, -1.0, -1.0, -1.0, -1.0, -1.0, -1.0, -1.0, -1.0, -1.0, -1.0, -1.0, -1.0, -1.0, -1.0, -1.0], [-1.0, -1.0, -1.0, -1.0, -1.0, -1.0, -1.0, -1.0, -1.0, -1.0, -1.0, -1.0, -1.0, -1.0, -1.0, -1.0, -1.0, -1.0, -1.0, -1.0, -1.0, -1.0, -1.0, -1.0, -1.0, -1.0, -1.0]], "Divider (kernel sum)"=sgl 10.0 ("Divider"), "error in (no error)"=w130, "Image Src"=w127) -> ("error out"=w140:errorcluster, "Image Dst Out"=w139:T8)  [unwired: 3 in, 3 out]
            n23 = case shown="\"Range 1\", Default" w111 {
              tunnel: ["Range 1 Templates - LEFT" "Range 0 Templates" "Range 2 Templates" "Range 3 Templates"] -> w171
              tunnel: [w541 w549 w561 w568] -> w169
              tunnel: [sgl 2.0 sgl 0.0 sgl 5.0 sgl 5.0] -> w168
              tunnel: [1 1 3 3] -> w167
              tunnel: [w538 w553 w557 w566] -> w113
              tunnel: "Correlation Score Threhsold" -> [w538 _ w557 w566]
              tunnel: "Correlation Score Threhsold (Range 0)" -> [_ w553 _ _]
              tunnel: [w536 w547 w555 w564] -> _
              tunnel: [w535 w545 w554 w563] -> w108
              frame "Range 1", Default {
                w543 = FALSE
                w542 = TRUE
                n24 = Unbundle By Name("Range 1 Default\nSetting Values") -> ("Max Scale Diff\nfrom Main"=w536:dbl, "Beacon Cushion (px)"=w535:dbl)
                n25 = Build Array(w542, w542, w543, w543, w543) -> (w541:bool[])
              }
              frame "Range 0" {
                (unwired) TRUE
                w550 = FALSE
                n26 = Unbundle By Name("Range 0 Default\nSetting Values") -> ("Max Scale Diff\nfrom Main"=w547:dbl, "Beacon Cushion (px)"=w545:dbl)
                n27 = Build Array(w550, w550, w550, w550, w550) -> (w549:bool[])
              }
              frame "Range 2" {
                (unwired) FALSE
                w562 = TRUE
                n28 = Unbundle By Name("Range 2 Default\nSetting Values") -> ("Max Scale Diff\nfrom Main"=w555:dbl, "Beacon Cushion (px)"=w554:dbl)
                n29 = Build Array(w562, w562, w562, w562, w562) -> (w561:bool[])
              }
              frame "Range 3" {
                (unwired) FALSE
                w569 = TRUE
                n30 = Unbundle By Name("Range 3 Default\nSetting Values") -> ("Max Scale Diff\nfrom Main"=w564:dbl, "Beacon Cushion (px)"=w563:dbl)
                n31 = Build Array(w569, w569, w569, w569, w569) -> (w568:bool[])
              }
            }
            n32 = Unbundle(w171) -> ("Sub - 2 File Path"=w124:path, "Sub Beacon Template File Path - ARRAY"=w170:path[])
            n33 = call "pattern_match_subvi.vi"("Match Image In"=w139, "Settings"=w123, "Template Image In"=w122, "select (false=mod))"="select (true= use advanced features\nfase= dont use)", "ROI Descriptor"=w125, "error in (no error)"=w140, "Path In"=w124) -> ("Refnum out"=w119:T8, "Number of Matches"=w120:i32, "Matches"=w121:T12[], "error out"=w118:errorcluster)  [unwired: 5 in]
            n34 = Equal?(x=w120, y=1) -> (x = y?=w176:bool)
            n35 = Array To Cluster(array=w121) -> (cluster=w175:T13)
            n36 = Unbundle By Name(w175) -> ("Matches[0].Correlation Score"=w174:sgl)
            "Current Correlation Score" <- w174
            n37 = Greater?(x=w174, y=w113) -> (0:w173:bool)
            n38 = And(x=w176, y=w173) -> (x .and. y?=w172:bool)
            n39 = case shown="True" w172 {
              tunnel: w119 -> [w648 w674]
              tunnel: w168 -> [_ w676]
              tunnel: w169 -> [_ w675]
              tunnel: w118 -> [_ w673]
              tunnel: w123 -> [_ w672]
              tunnel: [w653 w658] -> w183
              tunnel: [w652 w671] -> w182
              tunnel: [w652 w670] -> w181
              tunnel: [w652 w659] -> w180
              tunnel: [w652 w669] -> w225
              tunnel: [w651 w661] -> w220
              tunnel: [w651 w662] -> w219
              tunnel: [w648 w668] -> w189
              tunnel: [w649 w664] -> w110
              tunnel: w175 -> [_ w667]
              tunnel: w170 -> [_ w666]
              tunnel: w111 -> [_ w665]
              tunnel: [w645 w663] -> w109
              tunnel: w108 -> [_ w660]
              frame False {
                w650 = 0.0
                w651 = sgl 0.0 ("Scale")
                # "Don't Move servo"
                n40 = Bundle(w650, w650) -> (w649:cluster{dbl, dbl})  [unwired: 1 in]
                n41 = Bundle(159.0, 119.0) -> (w645:cluster{dbl, dbl})  [unwired: 1 in]
                n42 = Initialize Array(FALSE, 5 ("dimension size")) -> (w653:bool[])
                n43 = Initialize Array(0.0, 5 ("dimension size")) -> (w652:dbl[])
              }
              frame True {
                n44 = Unbundle By Name(w667) -> ("Matches[0].Position"=w664:cluster{"x":sgl, "y":sgl}, "Matches[0].Bounding Box"=w677:cluster{"x":sgl, "y":sgl}[], "Matches[0].Scale"=w661:sgl, "Matches[0].Score"=w662:sgl)
                n45 = case shown="\"Range 0\"" w665 {
                  tunnel: w677 -> [w709 _]
                  tunnel: w676 -> [w705 _]
                  tunnel: w675 -> [w693 _]
                  tunnel: w674 -> [w691 w764]
                  tunnel: w673 -> [w690 _]
                  tunnel: w672 -> [w689 _]
                  tunnel: [w687 w773] -> w658
                  tunnel: [w686 w767] -> w671
                  tunnel: [w685 w768] -> w670
                  tunnel: [w684 w769] -> w659
                  tunnel: [w683 w770] -> w669
                  tunnel: w661 -> [w682 _]
                  tunnel: [w681 w764] -> w668
                  tunnel: w666 -> [w680 _]
                  tunnel: w661 -> [_ w765]
                  tunnel: [w679 w761] -> w663
                  tunnel: w664 -> [w679 _]
                  tunnel: w660 -> [w678 _]
                  frame "Range 1", Default {
                    # "Build ROI for Individual Beacons Based on Main Bounding Box"
                    # "Starting X Lower Bound"
                    # "Beacons to Search For"
                    # "Length of\nIndividual Beacon ROI"
                    # "Length of Bounding Box"
                    # "Draw Bounding Box on Display Image"
                    n46 = Array To Cluster(array=w709) -> (cluster=w710:T14)
                    n47 = Unbundle By Name(w710) -> ("Bounding Box[0].x"=w703:sgl, "Bounding Box[0].y"=w700:sgl, "Bounding Box[2].x"=w706:sgl, "Bounding Box[2].y"=w699:sgl)
                    n48 = Bundle("x"=w703, "y"=w700, "x"=w706, "y"=w699) -> (w708:cluster{"x":sgl, "y":sgl, "x":sgl, "y":sgl})  [unwired: 1 in]
                    n49 = call "IMAQ Overlay Rectangle"("Rectangle"=w708, "Image"=w691) -> ("Image Out"=w688:T8)  [unwired: 8 in, 1 out]
                    n50 = Subtract(x=w706, y=w703) -> (x-y=w707:sgl)
                    n51 = Divide(x=w707, y=w705) -> (x/y=w704:sgl)
                    n52 = Multiply(x=w678, y=w682) -> (x*y=w701:dbl)
                    n53 = Divide(x=w701, y=sgl 100.0) -> (x/y=w696:dbl)
                    n54 = Subtract(x=w700, y=w696) -> (x-y=w698:dbl)
                    n55 = Add(x=w699, y=w696) -> (x+y=w697:dbl)
                    n56 = for {
                      N: 5 -> [_]
                      tunnel: w693 -> [w756] mode=indexing
                      shift-right: [w750] -> _
                      shift-left: w703 -> [w755]
                      tunnel: w704 -> [w754]
                      tunnel: w698 -> [w747]
                      tunnel: w697 -> [w746]
                      tunnel: [w753] -> w692 mode=indexing
                      tunnel: w696 -> [w748]
                      # "Divide Bounding Box"
                      # "Upper Bound of Current is\nLower Bound for Next"
                      n57 = case shown="True" w756 {
                        tunnel: w755 -> [w757 w758]
                        tunnel: w754 -> [_ w760]
                        tunnel: [w757 w759] -> w750
                        tunnel: [w757 w758] -> w752
                        frame False {
                          # "Don't Care"
                        }
                        frame True {
                          # "X Lower Bound"
                          n58 = Add(x=w758, y=w760) -> (x+y=w759:sgl)
                        }
                      }
                      n59 = Subtract(x=w752, y=w748) -> (x-y=w751:dbl)
                      n60 = Add(x=w750, y=w748) -> (x+y=w749:dbl)
                      n61 = call "Bound_RO_R_R0I.vi"("Bottom Right - Y"=w746, "Right - X"=w749, "Top Left - Y"=w747, "Top  Left - x"=w751) -> ("ROI Descriptor"=w753:T11)  [unwired: 7 in]
                    }
                    n62 = for {
                      N: 5 -> [_]
                      tunnel: w691 -> [w723]
                      tunnel: w690 -> [w722]
                      tunnel: w692 -> [w715] mode=indexing
                      tunnel: w680 -> [w721] mode=indexing
                      tunnel: [w720] -> w686 mode=indexing
                      tunnel: [w719] -> w685 mode=indexing
                      tunnel: [w718] -> w687 mode=indexing
                      tunnel: w693 -> [w717] mode=indexing
                      tunnel: w689 -> [w716]
                      shift-right: [w713] -> w681
                      shift-left: w688 -> [w714]
                      tunnel: [w712] -> w684 mode=indexing
                      tunnel: [w711] -> w683 mode=indexing
                      n63 = case shown="True" w717 {
                        tunnel: w723 -> [_ w738]
                        tunnel: w722 -> [_ w737]
                        tunnel: w715 -> [_ w736]
                        tunnel: w721 -> [_ w735]
                        tunnel: [w724 w731] -> w720
                        tunnel: [w724 w730] -> w719
                        tunnel: [FALSE w729] -> w718
                        tunnel: w716 -> [_ w728]
                        tunnel: [w724 w727] -> w712
                        tunnel: [w724 w726] -> w711
                        frame False {
                          w724 = sgl 0.0 ("x")
                        }
                        frame True {
                          n64 = call "Sub Beacon Pattern Match"("Image In"=w738, "ROI Descriptor (Geometric Matching 1)"=w736, "Settings (Geometric Matching 1)"=w728, "Template File Path (Geometric Matching 1)"=w735, "error in"=w737) -> ("Matches (Geometric Matching 1)"=w732:T12[], "Number of Matches (Geometric Matching 1)"=w733:i32)  [unwired: 19 in, 2 out]
                          n65 = Equal?(x=w733, y=1) -> (x = y?=w729:bool)
                          n66 = case shown="True" w729 {
                            tunnel: w732 -> [_ w744]
                            tunnel: [w739 w743] -> w731
                            tunnel: [w739 w742] -> w730
                            tunnel: [w739 w741] -> w727
                            tunnel: [w739 w740] -> w726
                            frame False {
                              w739 = sgl 0.0 ("x")
                            }
                            frame True {
                              n67 = Array To Cluster(array=w744) -> (cluster=w745:T15)
                              n68 = Unbundle By Name(w745) -> ("Matches (Geometric Matching 1)[0].Position.x"=w743:sgl, "Matches (Geometric Matching 1)[0].Position.y"=w742:sgl, "Matches (Geometric Matching 1)[0].Scale"=w741:sgl, "Matches (Geometric Matching 1)[0].Score"=w740:sgl)
                            }
                          }
                        }
                      }
                      n69 = call "IMAQ Overlay ROI"("ROI Descriptor"=w715, "Image"=w714) -> ("Image Out"=w713:T8)  [unwired: 8 in, 1 out]
                    }
                    "Horiztonall Beacon \nCushion (pixels)" <- w678
                  }
                  frame "Range 0" {
                    w766 = sgl 0.0
                    w772 = FALSE
                    # "Don't Move servo"
                    # "Insert Current Scale into index 0"
                    n70 = Bundle(159.0, 119.0) -> (w761:cluster{dbl, dbl})  [unwired: 1 in]
                    n71 = Build Array(TRUE, w772, w772, w772, w772) -> (w773:bool[])
                    n72 = Build Array(w765, w766, w766, w766, w766) -> (w769:sgl[])
                    n73 = Build Array(w766, w766, w766, w766, w766) -> (w768:sgl[])
                    n74 = Build Array(w766, w766, w766, w766, w766) -> (w770:sgl[])
                    n75 = Build Array(w766, w766, w766, w766, w766) -> (w767:sgl[])
                  }
                }
              }
            }
            "Beacons Found" <- w183
            "X Coordinates" <- w182
            "Y Coordinates" <- w181
            "Beacon - Scales" <- w180
            "beacon - Scores" <- w225
            "Current  Scale" <- w220
            "Current  Score" <- w219
            n76 = shared-variable "RT myRIO Target - Overlord\\Localization_Variables_r0.lvlib\\LEFT_BEACON_BOOL_array"(w183) -> ()  [unwired: 1 in, 1 out]
            n77 = shared-variable "RT myRIO Target - Overlord\\Localization_Variables_r0.lvlib\\LEFT_BEACON_X_array"(w182) -> ()  [unwired: 1 in, 1 out]
            n78 = shared-variable "RT myRIO Target - Overlord\\Localization_Variables_r0.lvlib\\LEFT_BEACON_Y_array"(w181) -> ()  [unwired: 1 in, 1 out]
            n79 = shared-variable "RT myRIO Target - Overlord\\Localization_Variables_r0.lvlib\\LEFT_BEACON_Scales"(w180) -> ()  [unwired: 1 in, 1 out]
            n80 = Boolean To (0,1)(Boolean=w183) -> (0, 1=w227:i16[])
            n81 = Add Array Elements(numeric array=w227) -> (sum=w226:i16)
            n82 = Greater Or Equal?(x=w226, y=w167) -> (x >= y?=w158:bool)
            "Current Valid?" <- w158
            n83 = local read "History Size"() -> (w211:i32)
            n84 = Decrement(x=w211) -> (x-1=w224:i32)
            n85 = for {
              N: w211 -> [_]
              shift-right: [w623] -> w178
              shift-left: w223 -> [w611]
              tunnel: w224 -> [w619]
              shift-right: [w616] -> w147
              shift-left: w222 -> [w618]
              shift-right: [w615] -> w177
              shift-left: w221 -> [w617]
              tunnel: w220 -> [w614]
              tunnel: w219 -> [w613]
              tunnel: w158 -> [w612]
              i -> [w622]
              # "Reverse Index"
              n86 = Subtract(x=w619, y=w622) -> (x-y=w620:i32)
              n87 = Equal To 0?(x=w620) -> (x = 0?=w621:bool)
              n88 = case shown="True" w621 {
                tunnel: w620 -> [w624 w643]
                tunnel: w611 -> [w634 w636]
                tunnel: [w632 w635] -> w623
                tunnel: w612 -> [_ w644]
                tunnel: w618 -> [w629 w642]
                tunnel: w617 -> [w628 w641]
                tunnel: [w627 w639] -> w616
                tunnel: [w626 w640] -> w615
                tunnel: w614 -> [_ w638]
                tunnel: w613 -> [_ w637]
                frame False {
                  # "Shift Old"
                  n89 = Decrement(x=w624) -> (x-1=w625:i32)
                  n90 = Index Array(array=w634, index=w625) -> (element=w633:bool)
                  n91 = Index Array(array=w629, index=w625) -> (element=w631:dbl)
                  n92 = Index Array(array=w628, index=w625) -> (element=w630:dbl)
                  n93 = Replace Array Subset(array=w634, new element=w633, index=w624) -> (w632:bool[])
                  n94 = Replace Array Subset(array=w629, new element=w631, index=w624) -> (w627:dbl[])
                  n95 = Replace Array Subset(array=w628, new element=w630, index=w624) -> (w626:dbl[])
                }
                frame True {
                  # "Score"
                  # "Scale"
                  # "Valid"
                  # "insert New"
                  n96 = Replace Array Subset(array=w642, new element=w638, index=w643) -> (w639:dbl[])
                  n97 = Replace Array Subset(array=w641, new element=w637, index=w643) -> (w640:dbl[])
                  n98 = Replace Array Subset(array=w636, new element=w644, index=w643) -> (w635:bool[])
                }
              }
            }
            n99 = Boolean To (0,1)(Boolean=w178) -> (0, 1=w217:i16[])
            n100 = Add Array Elements(numeric array=w217) -> (sum=w216:i16)
            n101 = Greater Or Equal?(x=w216, y="Valid Treshold\nfor Lock") -> (x >= y?=w145:bool)
            "Lock Status" <- w145
            n102 = shared-variable "RT myRIO Target - Overlord\\Localization_Variables_r0.lvlib\\Image Lock - L"(w145) -> ()  [unwired: 1 in, 1 out]
            n103 = Initialize Array(u8 0, "Max Window\n for Avg") -> (w214:u8[])
            n104 = while {
              shift-right: [w594] -> w210
              shift-left: w214 -> [w596]
              tunnel: w178 -> [w602] mode=indexing
              shift-right: [w600] -> w207
              shift-left: u8 0 -> [w603]
              tunnel: w211 -> [w601]
              tunnel: "Max Window\n for Avg" -> [w593]
              i -> [w595]
              stop <- w597 stop-if-true
              # "Grab Last 'X' Valid Indexes"
              n105 = case shown="True" w602 {
                tunnel: w603 -> [w605 w607]
                tunnel: [w605 w610] -> w600
                tunnel: w596 -> [w604 w609]
                tunnel: w595 -> [_ w608]
                tunnel: [w604 w606] -> w594
                frame False {
                }
                frame True {
                  # "Update Index\nto use"
                  # "Increment\nValid Count"
                  n106 = Replace Array Subset(array=w609, new element=w608, index=w607) -> (w606:u8[])
                  n107 = Increment(x=w607) -> (x+1=w610:u8)
                }
              }
              n108 = Greater?(x=w595, y=w601) -> (0:w598:bool)
              n109 = Greater Or Equal?(x=w600, y=w593) -> (x >= y?=w599:bool)
              n110 = Or(x=w599, y=w598) -> (x .or. y?=w597:bool)
            }
            n111 = Greater Or Equal?(x=w207, y=u8 2) -> (x >= y?=w208:bool)
            n112 = case shown="True" w208 {
              tunnel: w207 -> [_ w577]
              tunnel: w210 -> [_ w583]
              tunnel: w147 -> [_ w582]
              tunnel: w177 -> [_ w581]
              tunnel: ["Avg Scale - Last" w575] -> w166
              tunnel: ["Avg Score - Last" w574] -> w165
              frame False {
              }
              frame True {
                w580 = 0.0
                n113 = for {
                  N: w577 -> [_]
                  tunnel: w583 -> [w590] mode=indexing
                  tunnel: w582 -> [w592]
                  tunnel: w581 -> [w591]
                  shift-right: [w588] -> w579
                  shift-left: w580 -> [w586]
                  shift-right: [w589] -> w578
                  shift-left: w580 -> [w585]
                  # "Fetch Last Valid Values"
                  n114 = Index Array(array=w592, index=w590) -> (element=w587:dbl)
                  n115 = Index Array(array=w591, index=w590) -> (element=w584:dbl)
                  n116 = Add(x=w587, y=w586) -> (x+y=w588:dbl)
                  n117 = Add(x=w584, y=w585) -> (x+y=w589:dbl)
                }
                n118 = To Double Precision Float(number=w577) -> (double precision float=w576:dbl)
                n119 = Divide(x=w579, y=w576) -> (x/y=w575:dbl)
                n120 = Divide(x=w578, y=w576) -> (x/y=w574:dbl)
                n121 = local write "Avg Scale - Last"(w575) -> ()
                n122 = local write "Avg Score - Last"(w574) -> ()
              }
            }
            "Avg Score" <- w165
            "Avg Scale" <- w166
            n123 = And(x=w145, y=w144) -> (x .and. y?=w146:bool)
            n124 = case shown="False" w146 {
              selector: w146 -> [_ w231]
              tunnel: [w229 w230] -> w143
              tunnel: w144 -> [w229 _]
              frame False {
              }
              frame True {
                # "Pull Down Start Up \nFlag"
                n125 = Not(x=w231) -> (.not. x?=w230:bool)
              }
            }
            n126 = Unbundle By Name(w123) -> ("Minimum Match Score"=w163:sgl, "Range Settings"=w194:T6[], "Curve Parameters"=w160:T5)
            n127 = Index Array(array=w194, index=u32 1) -> (element=w195:T6)
            n128 = Unbundle(w195) -> ("Min"=w162:dbl, "Max"=w161:dbl)  [unwired: 1 out]
            n129 = case shown="False" w143 {
              tunnel: w145 -> [w254 _]
              tunnel: w111 -> [w253 w534]
              tunnel: w166 -> [w252 _]
              tunnel: [w236 w534] -> _
              tunnel: w166 -> [w251 _]
              tunnel: w165 -> [w250 _]
              tunnel: "Score\nCushion" -> [w249 _]
              tunnel: w163 -> [w248 w531]
              tunnel: w162 -> [w247 w530]
              tunnel: w161 -> [w246 w529]
              tunnel: w110 -> [w245 _]
              tunnel: w125 -> [w244 w533]
              tunnel: w160 -> [w243 _]
              tunnel: w160 -> [w242 w532]
              tunnel: [w241 w531] -> w152
              tunnel: [w240 w530] -> w150
              tunnel: [w239 w529] -> w151
              tunnel: [w238 w533] -> w149
              tunnel: [w237 w532] -> w157
              tunnel: [w235 FALSE] -> w159
              tunnel: w158 -> [w234 _]
              tunnel: w147 -> [w233 w527]
              tunnel: [w232 w527] -> w148
              frame False {
                # "Current Template"
                # "Image Lock?"
                n130 = case shown="False" w254 {
                  tunnel: w253 -> [_ w326]
                  tunnel: [w255 w289] -> w236
                  tunnel: w252 -> [_ w327]
                  tunnel: w251 -> [_ w325]
                  tunnel: w250 -> [_ w323]
                  tunnel: w249 -> [_ w322]
                  tunnel: w248 -> [_ w321]
                  tunnel: w247 -> [_ w320]
                  tunnel: w246 -> [_ w319]
                  tunnel: w245 -> [_ w318]
                  tunnel: w244 -> [_ w317]
                  tunnel: w243 -> [_ w314]
                  tunnel: w242 -> [w260 w299]
                  tunnel: [w259 w294] -> w237
                  tunnel: [w271 w293] -> w238
                  tunnel: [w280 w292] -> w241
                  tunnel: [w279 w291] -> w240
                  tunnel: [w278 w290] -> w239
                  tunnel: [FALSE w288] -> w235
                  tunnel: w234 -> [_ w287]
                  tunnel: w233 -> [w257 w286]
                  tunnel: [w257 w285] -> w232
                  frame False {
                    w255 = T3."Range 0" ("Current Template")
                    # "Apply default settings for the selected template"
                    # "Initial ROI Descriptor"
                    # "Check Other Camera?"
                    n131 = case shown="\"Range 0\"" w255 {
                      tunnel: [w281 w282 w283 w284] -> w256
                      frame "Range 1", Default {
                        n132 = local read "Range 1 Default\nSetting Values"() -> (w281:T1)
                      }
                      frame "Range 2" {
                        n133 = local read "Range 2 Default\nSetting Values"() -> (w282:T1)
                      }
                      frame "Range 3" {
                        n134 = local read "Range 3 Default\nSetting Values"() -> (w283:T1)
                      }
                      frame "Range 0" {
                        n135 = local read "Range 0 Default\nSetting Values"() -> (w284:T1)
                      }
                    }
                    n136 = Unbundle By Name(w256) -> ("Min Score"=w280:dbl, "Min Scale"=w279:dbl, "Max Scale"=w278:dbl, "Curve Parameters"=w261:T16)
                    n137 = Bundle(0, 0, 640, 480, 0) -> (w277:cluster{i32, i32, i32, i32, i32})  [unwired: 1 in]
                    n138 = call "IMAQ Convert Rectangle to ROI"("Rectangle"=w277) -> ("ROI Descriptor"=w271:T11)  [unwired: 8 in, 1 out]
                    n139 = Unbundle By Name(w261) -> ("Min Length"=w265:i32, "Row Search Step"=w266:i32, "Col Search Step"=w267:i32)
                    n140 = Unbundle(w260) -> ("Extraction Mode"=w262:u32, "Edge Threshold"=w263:i32, "Edge Filter Size"=w264:u32, "Max Endpoint Gap"=w268:i32, "Closed"=w269:bool, "Subpixel"=w270:bool)  [unwired: 3 out]
                    n141 = Bundle("Extraction Mode"=w262, "Edge Threshold"=w263, "Edge Filter Size"=w264, "Min Length"=w265, "Row Search Step"=w266, "Col Search Step"=w267, "Max Endpoint Gap"=w268, "Closed"=w269, "Subpixel"=w270) -> (w259:T17)  [unwired: 1 in]
                  }
                  frame True {
                    # "Update Search Settings"
                    # "Next State"
                    # "Changing Templates?"
                    # "Update Template"
                    n142 = case shown="\"Range 1\", Default" w326 {
                      selector: w326 -> [w459 w490 w508 w523]
                      tunnel: w327 -> [w460 w492 w509 w524]
                      tunnel: [w461 w491 w507 w522] -> w289
                      tunnel: [w475 w481 w501 w516] -> w324
                      tunnel: [w474 w480 w500 w515] -> w316
                      tunnel: [w473 w479 w499 w514] -> w315
                      tunnel: [w472 w482 w505 w520] -> w310
                      tunnel: [w471 w484 w502 w517] -> w302
                      tunnel: [w470 w485 w503 w518] -> w301
                      tunnel: [w469 w488 w504 w519] -> w300
                      frame "Range 1", Default {
                        # "Next Template"
                        # "Next Template"
                        n143 = local read "Range 1 Default\nSetting Values"() -> (w476:T1)
                        n144 = Unbundle By Name(w476) -> ("Lower Transition Scale"=w457:sgl, "Upper Transition Scale"=w458:sgl, "ROI Vertical"=w473:dbl, "ROI Horizontal"=w474:dbl, "Scale Cushion"=w475:dbl, "Curve Parameters"=w472:T16, "Min Score"=w471:dbl, "Min Scale"=w470:dbl, "Max Scale"=w469:dbl)
                        n145 = Less?(x=w460, y=w457) -> (x < y?=w468:bool)
                        n146 = Not(x=w468) -> (.not. x?=w467:bool)
                        n147 = Select(t=w459, s=w467, f=T3."Range 2" ("Initial Template 2")) -> (s? t:f=w464:T3)
                        n148 = Greater?(x=w460, y=w458) -> (0:w466:bool)
                        n149 = Not(x=w466) -> (.not. x?=w465:bool)
                        n150 = Select(t=w464, s=w465, f=T3."Range 0" ("Initial Template 2")) -> (s? t:f=w461:T3)
                      }
                      frame "Range 2" {
                        # "Next Template"
                        # "Next Template"
                        n151 = local read "Range 2 Default\nSetting Values"() -> (w489:T1)
                        n152 = Unbundle By Name(w489) -> ("Lower Transition Scale"=w487:sgl, "Upper Transition Scale"=w486:sgl, "ROI Vertical"=w479:dbl, "ROI Horizontal"=w480:dbl, "Scale Cushion"=w481:dbl, "Curve Parameters"=w482:T16, "Min Score"=w484:dbl, "Min Scale"=w485:dbl, "Max Scale"=w488:dbl)
                        n153 = Less?(x=w492, y=w487) -> (x < y?=w496:bool)
                        n154 = Not(x=w496) -> (.not. x?=w495:bool)
                        n155 = Select(t=w490, s=w495, f=T3."Range 3" ("Initial Template 2")) -> (s? t:f=w483:T3)
                        n156 = Greater?(x=w492, y=w486) -> (0:w494:bool)
                        n157 = Not(x=w494) -> (.not. x?=w493:bool)
                        n158 = Select(t=w483, s=w493, f=T3."Range 1" ("Initial Template 2")) -> (s? t:f=w491:T3)
                      }
                      frame "Range 3" {
                        # "Next Template"
                        n159 = local read "Range 3 Default\nSetting Values"() -> (w506:T1)
                        n160 = Unbundle By Name(w506) -> ("Upper Transition Scale"=w498:sgl, "ROI Vertical"=w499:dbl, "ROI Horizontal"=w500:dbl, "Scale Cushion"=w501:dbl, "Curve Parameters"=w505:T16, "Min Score"=w502:dbl, "Min Scale"=w503:dbl, "Max Scale"=w504:dbl)  [unwired: 1 out]
                        n161 = Greater?(x=w509, y=w498) -> (0:w511:bool)
                        n162 = Not(x=w511) -> (.not. x?=w510:bool)
                        n163 = Select(t=w508, s=w510, f=T3."Range 2" ("Initial Template 2")) -> (s? t:f=w507:T3)
                      }
                      frame "Range 0" {
                        # "Next Template"
                        n164 = local read "Range 0 Default\nSetting Values"() -> (w521:T1)
                        n165 = Unbundle By Name(w521) -> ("Lower Transition Scale"=w512:sgl, "ROI Vertical"=w514:dbl, "ROI Horizontal"=w515:dbl, "Scale Cushion"=w516:dbl, "Curve Parameters"=w520:T16, "Min Score"=w517:dbl, "Min Scale"=w518:dbl, "Max Scale"=w519:dbl)  [unwired: 1 out]
                        n166 = Less?(x=w524, y=w512) -> (x < y?=w526:bool)
                        n167 = Not(x=w526) -> (.not. x?=w525:bool)
                        n168 = Select(t=w523, s=w525, f=T3."Range 1" ("Initial Template 2")) -> (s? t:f=w522:T3)
                      }
                    }
                    n169 = Unbundle By Name(w310) -> ("Min Length"=w309:i32, "Row Search Step"=w308:i32, "Col Search Step"=w307:i32)
                    n170 = Unbundle(w314) -> ("Extraction Mode"=w313:u32, "Edge Threshold"=w312:i32, "Edge Filter Size"=w311:u32, "Max Endpoint Gap"=w306:i32, "Closed"=w305:bool, "Subpixel"=w304:bool)  [unwired: 3 out]
                    n171 = Bundle("Extraction Mode"=w313, "Edge Threshold"=w312, "Edge Filter Size"=w311, "Min Length"=w309, "Row Search Step"=w308, "Col Search Step"=w307, "Max Endpoint Gap"=w306, "Closed"=w305, "Subpixel"=w304) -> (w303:T17)  [unwired: 1 in]
                    n172 = Not Equal?(x=w289, y=w326) -> (x != y?=w288:bool)
                    n173 = case shown="True" w288 {
                      tunnel: w287 -> [w350 _]
                      tunnel: w325 -> [w349 _]
                      tunnel: w324 -> [w348 _]
                      tunnel: w323 -> [w347 _]
                      tunnel: w322 -> [w346 _]
                      tunnel: w321 -> [w345 _]
                      tunnel: w320 -> [w344 _]
                      tunnel: w319 -> [w343 _]
                      tunnel: w318 -> [w342 _]
                      tunnel: w317 -> [w341 _]
                      tunnel: w316 -> [w340 _]
                      tunnel: w315 -> [w339 _]
                      tunnel: [w337 w424] -> w292
                      tunnel: w303 -> [w328 _]
                      tunnel: [w336 w423] -> w291
                      tunnel: [w335 w422] -> w290
                      tunnel: w302 -> [_ _]
                      tunnel: w301 -> [_ _]
                      tunnel: w300 -> [_ _]
                      tunnel: w289 -> [_ w426]
                      tunnel: w299 -> [_ w439]
                      tunnel: [w329 w438] -> w294
                      tunnel: [w334 w433] -> w298
                      tunnel: [w333 w432] -> w297
                      tunnel: [w332 w415] -> w296
                      tunnel: [w331 w416] -> w295
                      tunnel: w286 -> [w330 w418]
                      tunnel: [w330 w417] -> w285
                      frame False {
                        w338 = 500.0 ("y")
                        # "Current Valid?"
                        # "********"
                        # "Apply Limit to Score"
                        # "Score out"
                        # "Apply Limits to ROI"
                        n174 = case shown="False" w350 {
                          tunnel: w347 -> [_ w399]
                          tunnel: w346 -> [_ w398]
                          tunnel: w349 -> [_ w389]
                          tunnel: w348 -> [w378 w397]
                          tunnel: [w361 w392] -> w334
                          tunnel: [w360 w388] -> w333
                          tunnel: [w359 w391] -> w332
                          tunnel: [w358 w390] -> w331
                          tunnel: [w374 w387] -> w351
                          tunnel: [w373 w386] -> w336
                          tunnel: [w372 w385] -> w335
                          tunnel: w341 -> [w370 _]
                          tunnel: w345 -> [w357 _]
                          tunnel: w344 -> [w356 _]
                          tunnel: w343 -> [w355 _]
                          tunnel: w342 -> [_ w384]
                          tunnel: w340 -> [_ w380]
                          tunnel: w339 -> [_ w381]
                          tunnel: [w353 w379] -> w329
                          tunnel: w328 -> [w353 w379]
                          frame False {
                            # "Current Match was Invalid"
                            n175 = Divide(x=w378, y=sgl 3.0) -> (x/y=w376:dbl)
                            n176 = Subtract(x=w356, y=w376) -> (x-y=w373:dbl)
                            n177 = Add(x=w355, y=w376) -> (x+y=w372:dbl)
                            n178 = Subtract(x=w357, y="Score Decay \nFactor 2") -> (x-y=w374:dbl)
                            n179 = call "IMAQ Convert ROI to Rectangle"("ROI Descriptor"=w370) -> ("Rectangle"=w371:T18)  [unwired: 8 in, 1 out]
                            n180 = Unbundle By Name(w371) -> ("Left"=w365:i32, "Top"=w364:i32, "Right"=w363:i32, "Bottom"=w362:i32)
                            n181 = To Long Integer(number="ROI Decay Factor (px)") -> (32bit integer=w367:i32)
                            n182 = Divide(x="ROI Decay Factor (px)", y=sgl 10.0) -> (x/y=w369:dbl)
                            n183 = Subtract(x=w365, y=w367) -> (x-y=w361:i32)
                            n184 = Add(x=w363, y=w367) -> (x+y=w359:i32)
                            n185 = To Long Integer(number=w369) -> (32bit integer=w366:i32)
                            n186 = Subtract(x=w364, y=w366) -> (x-y=w360:i32)
                            n187 = Add(x=w362, y=w366) -> (x+y=w358:i32)
                          }
                          frame True {
                            (unwired) sgl 109.0 ("x")
                            (unwired) sgl 159.0 ("x")
                            # "Current Match was Valid"
                            # "Center of Image"
                            # "Main ROI"
                            # "Horizontal Scale \n(smaller number = smaller ROI)"
                            n188 = Subtract(x=w399, y=w398) -> (x-y=w387:dbl)
                            n189 = case shown="0, Default" "ROBOT STATE\n(fwd, bwd, neither) 2" {
                              tunnel: w389 -> [w404 w409 w414]
                              tunnel: [w403 w405 w410] -> w385
                              tunnel: w397 -> [w401 w408 w413]
                              tunnel: [w402 w406 w411] -> w386
                              frame 0, Default {
                                n190 = Subtract(x=w404, y=w401) -> (x-y=w402:dbl)
                                n191 = Add(x=w401, y=w404) -> (x+y=w403:dbl)
                              }
                              frame 1 {
                                n192 = Subtract(x=w409, y=5.0) -> (x-y=w406:dbl)
                                n193 = Add(x=w408, y=w409) -> (x+y=w405:dbl)
                              }
                              frame -1 {
                                n194 = Subtract(x=w414, y=w413) -> (x-y=w411:dbl)
                                n195 = Add(x=5.0 ("y"), y=w414) -> (x+y=w410:dbl)
                              }
                            }
                            n196 = Unbundle(w384) -> ("x"=w383:dbl, "y"=w382:dbl)
                            n197 = Divide(x=w389, y=w381) -> (x/y=w395:dbl)
                            n198 = Multiply(x=w389, y=w380) -> (x*y=w393:dbl)
                            n199 = Divide(x=w393, y=sgl 2.0) -> (x/y=w396:dbl)
                            n200 = Add(x=w382, y=w395) -> (x+y=w390:dbl)
                            n201 = Subtract(x=w382, y=w395) -> (x-y=w388:dbl)
                            n202 = Subtract(x=w383, y=w396) -> (x-y=w392:dbl)
                            n203 = Add(x=w396, y=w383) -> (x+y=w391:dbl)
                          }
                        }
                        n204 = Greater?(x=w351, y=w338) -> (0:w352:bool)
                        n205 = Select(t=w351, s=w352, f=w338) -> (s? t:f=w337:dbl)
                      }
                      frame True {
                        w419 = 80.0 ("Avg Scale - Last")
                        w429 = sgl 125.0 ("x")
                        w430 = sgl 109.0 ("x")
                        w431 = sgl 159.0 ("x")
                        # "Reset Scale to 100"
                        # "\"Start Scale\""
                        # "Center of Image"
                        # "Main ROI"
                        # "Horizontal Scale \n(smaller number = smaller ROI)"
                        # "Apply New Curve Parameters"
                        # "Next State"
                        # "Changing States - Apply Initial Settings for that State"
                        n206 = local read "History Size"() -> (w420:i32)
                        n207 = case shown="\"Range 1\", Default" w426 {
                          tunnel: [w453 w454 w455 w456] -> w425
                          frame "Range 1", Default {
                            n208 = local read "Range 1 Default\nSetting Values"() -> (w453:T1)
                          }
                          frame "Range 2" {
                            n209 = local read "Range 2 Default\nSetting Values"() -> (w454:T1)
                          }
                          frame "Range 3" {
                            n210 = local read "Range 3 Default\nSetting Values"() -> (w455:T1)
                          }
                          frame "Range 0" {
                            n211 = local read "Range 0 Default\nSetting Values"() -> (w456:T1)
                          }
                        }
                        n212 = local write "Avg Scale - Last"(w419) -> ()
                        n213 = for {
                          N: w420 -> [_]
                          tunnel: w419 -> [w450]
                          shift-right: [w449] -> w417
                          shift-left: w418 -> [w452]
                          i -> [w451]
                          n214 = Replace Array Subset(array=w452, new element=w450, index=w451) -> (w449:dbl[])
                        }
                        n215 = Unbundle By Name(w425) -> ("Min Score"=w424:dbl, "Min Scale"=w423:dbl, "Max Scale"=w422:dbl, "Curve Parameters"=w421:T16, "ROI Vertical"=w428:dbl, "ROI Horizontal"=w427:dbl)
                        n216 = Unbundle By Name(w421) -> ("Min Length"=w443:i32, "Row Search Step"=w444:i32, "Col Search Step"=w445:i32)
                        n217 = Unbundle(w439) -> ("Extraction Mode"=w440:u32, "Edge Threshold"=w441:i32, "Edge Filter Size"=w442:u32, "Max Endpoint Gap"=w446:i32, "Closed"=w447:bool, "Subpixel"=w448:bool)  [unwired: 3 out]
                        n218 = Bundle("Extraction Mode"=w440, "Edge Threshold"=w441, "Edge Filter Size"=w442, "Min Length"=w443, "Row Search Step"=w444, "Col Search Step"=w445, "Max Endpoint Gap"=w446, "Closed"=w447, "Subpixel"=w448) -> (w438:T17)  [unwired: 1 in]
                        n219 = Divide(x=w429, y=w428) -> (x/y=w436:dbl)
                        n220 = Multiply(x=w429, y=w427) -> (x*y=w434:dbl)
                        n221 = Divide(x=w434, y=sgl 2.0) -> (x/y=w437:dbl)
                        n222 = Add(x=w430, y=w436) -> (x+y=w416:dbl)
                        n223 = Subtract(x=w430, y=w436) -> (x-y=w432:dbl)
                        n224 = Subtract(x=w431, y=w437) -> (x-y=w433:dbl)
                        n225 = Add(x=w437, y=w431) -> (x+y=w415:dbl)
                      }
                    }
                    n226 = call "Bound_RO_R_R0I.vi"("Bottom Right - Y"=w295, "Right - X"=w296, "Top Left - Y"=w297, "Top  Left - x"=w298) -> ("ROI Descriptor"=w293:T11)  [unwired: 7 in]
                  }
                }
              }
              frame True {
              }
            }
            n227 = Less?(x=w152, y="Absolute\nMinimum Score") -> (x < y?=w200:bool)
            n228 = Less?(x=w150, y="Absolute\nMinimum Scale") -> (x < y?=w203:bool)
            n229 = Greater?(x=w151, y="Absolute\nMaximum Scale") -> (0:w206:bool)
            n230 = Greater?(x=w150, y=w151) -> (0:w202:bool)
            n231 = Less?(x=w151, y=w150) -> (x < y?=w205:bool)
            n232 = Select(t="Absolute\nMinimum Score", s=w200, f=w152) -> (s? t:f=w188:dbl)
            "New Min Score" <- w188
            n233 = Or(x=w203, y=w202) -> (x .or. y?=w201:bool)
            n234 = Or(x=w206, y=w205) -> (x .or. y?=w204:bool)
            n235 = Select(t="Absolute\nMinimum Scale", s=w201, f=w150) -> (s? t:f=w187:dbl)
            "New Low Scale" <- w187
            n236 = Select(t="Absolute\nMaximum Scale", s=w204, f=w151) -> (s? t:f=w186:dbl)
            "New high Scale" <- w186
            n237 = Bundle("index"=w193, "Min"=w187, "Max"=w186) -> (w192:cluster{"index":u32, "Min":dbl, "Max":dbl})  [unwired: 1 in]
            n238 = Replace Array Subset(array=w194, new element=w192, index=w193) -> (w191:T6[])
            n239 = Bundle By Name(cluster=w123, "Minimum Match Score"=w188, "Range Settings"=w191, "Curve Parameters"=w157) -> (w190:T7)
            n240 = call "IMAQ Overlay ROI"("ROI Descriptor"=w149, "Image"=w189) -> ("Image Out"=→"Right Image out":T8)  [unwired: 8 in, 1 out]
            n241 = Unbundle By Name(w157) -> ("Min Length"=w156:i32, "Row Search Step Size"=w155:i32, "Col Search Step Size"=w154:i32)
            n242 = Bundle("Min Length"=w156, "Row Search Step Size"=w155, "Col Search Step Size"=w154) -> (w153:T19)  [unwired: 1 in]
            n243 = Bundle("Min Score"=w188, "Min"=w187, "Max"=w186, w153) -> (w185:T20)  [unwired: 1 in]
            n244 = case shown="True" w159 {
              tunnel: w109 -> [w776 w782]
              tunnel: w158 -> [w777 w788]
              tunnel: w183 -> [_ _]
              tunnel: w185 -> [w779 w786]
              tunnel: w145 -> [w778 w789]
              tunnel: w107 -> [w775 w787]
              tunnel: [w774 w785] -> w142
              frame False {
                n245 = Bundle(w778, w777, "Initial Template"=w775, "Position"=w776, w779) -> (w774:T21)  [unwired: 1 in]
              }
              frame True {
                # "Check if Tracking is Available for the Next Template State"
                n246 = local read "Current Template"() -> (w780:T3)
                n247 = Unbundle(w782) -> ("x"=w784:dbl, "y"=w783:dbl)
                n248 = case shown="\"Range 1\"" w787 {
                  tunnel: w784 -> [w794 w803 _ _]
                  tunnel: w783 -> [w790 w802 _ _]
                  tunnel: w782 -> [_ w800 w811 _]
                  tunnel: [w793 w801 w811 w814] -> w781
                  tunnel: w780 -> [w791 w799 _ _]
                  frame "Range 1" {
                    n249 = case shown="\"Range 2\"" w791 {
                      tunnel: w794 -> [w795 w798]
                      tunnel: [w795 w796] -> w792
                      frame "Range 0", Default {
                      }
                      frame "Range 2" {
                        n250 = Add(x=w798, y=-70.0) -> (x+y=w796:dbl)
                      }
                    }
                    n251 = Bundle("x"=w792, "y"=w790) -> (w793:cluster{"x":dbl, "y":dbl})  [unwired: 1 in]
                  }
                  frame "Range 2" {
                    # "Depends on Current State"
                    n252 = case shown="\"Range 3\"" w799 {
                      tunnel: w803 -> [w808 _ _]
                      tunnel: w802 -> [w805 _ _]
                      tunnel: [w804 w809 w810] -> w801
                      tunnel: w800 -> [_ w809 w810]
                      frame "Range 1" {
                        n253 = Add(x=w808, y=70.0) -> (x+y=w806:dbl)
                        n254 = Bundle(w806, "y"=w805) -> (w804:cluster{dbl, "y":dbl})  [unwired: 1 in]
                      }
                      frame "Range 2", Default {
                      }
                      frame "Range 3" {
                      }
                    }
                  }
                  frame "Range 3", Default {
                  }
                  frame "Range 0" {
                    # "Don't Move servo"
                    n255 = Bundle(159.0, 119.0) -> (w814:cluster{dbl, dbl})  [unwired: 1 in]
                  }
                }
                n256 = Bundle(w789, w788, "Initial Template"=w787, "Position"=w781, w786) -> (w785:T21)  [unwired: 1 in]
              }
            }
            "Tracking Info" <- w142
            n257 = shared-variable "RT myRIO Target - Overlord\\Localization_Variables_r0.lvlib\\Info - Left"(w142) -> ()  [unwired: 1 in, 1 out]
            "Next Template" <- w107
          }
          frame #2 {
            n258 = shared-variable "RT myRIO Target - Overlord\\Localization_Variables_r0.lvlib\\Left Servo Angle_Image"(w817) -> ()  [unwired: 1 in, 1 out]
            n259 = shared-variable "RT myRIO Target - Overlord\\Localization_Variables_r0.lvlib\\Left_Flag"(TRUE ("RIGHT_FLAG")) -> ()  [unwired: 1 in, 1 out]
          }
        }
        "Startup Flag" <- w75
        "Valid Scale History" <- w82
        "Valid Beacon History - in" <- w84
        "Valid Score History" <- w81
        "Current Search Settings" <- w92
        "Current Template" <- w79
      }
    }
    frame #2 {
      n260 = call <vilib>:"IMAQdx Close Camera.vi"("Session In"=w819) -> ()  [unwired: 10 in, 1 out]
    }
  }
